vi "Dashboard Main20170221.vi"() -> ()   [LabVIEW 2016]
uses:
  <vilib>/Utility/miscctls.llb/LVRangeTypeDef.ctl
  <vilib>/Platform/TimedLoop/XDataNode/timing_clust.ctl
  <vilib>/Platform/TimedLoop/XDataNode/nitl_modes.ctl
  <vilib>/Platform/TimedLoop/XDataNode/wakeup.ctl
  <vilib>/Utility/miscctls.llb/LVRowAndColumnTypeDef.ctl
  <vilib>/event_ctls.llb/eventvkey.ctl
  <vilib>/Rock Robotics/WPI/Dashboard/WPI_DashboardLogging Global.vi
  <vilib>/Rock Robotics/Network Tables/NT Read Numeric Array.vi
  <vilib>/Rock Robotics/Network Tables/NT Write Boolean.vi
  <vilib>/platform/TimedLoop/XDataNode/XDataNode.xnode
  <vilib>/Platform/TimedLoop/XDataNode/XDNodeRunTimeDep.lvlib
panel:
  in  "Camera Tab":T1(tab)
  out "Image Message":string="Timeout in Camera Communications"
  in  "Camera Settings 1":T2={"Frame Rate"=30, "Compression"=30, "Size"=1, "DB Camera Config"=FALSE} {"Frame Rate" scale=1.0..30.0; "Compression" scale=100.0..-1.0; "Size" items=["640x480", "320x240", "160x120"]}
  out "Dashboard Image 1":T3(plugin-control)
  out "Camera Info 1":cluster{"Mbps LED":bool, "Mbps":dbl, "fps":dbl} {"fps" format="%#.1g"; "Mbps" format="%#.1g"}
  in  "Camera Name 1":string(combo)="No Camera Selection"
  out "Image Message 2":string="Timeout in Camera Communications"
  in  "Camera Settings 2":T2={"Frame Rate"=30, "Compression"=30, "Size"=1, "DB Camera Config"=FALSE} {"Frame Rate" scale=1.0..30.0; "Compression" scale=100.0..-1.0; "Size" items=["640x480", "320x240", "160x120"]}
  out "Dashboard Image 2":T3(plugin-control)
  out "Camera Info 2":cluster{"Mbps LED":bool, "Mbps":dbl, "fps":dbl} {"fps" format="%#.1g"; "Mbps" format="%#.1g"}
  in  "Camera Name 2":string(combo)="No Camera Selection"
  out "Image Message 3":string="Timeout in Camera Communications"
  in  "Camera Settings 3":T2={"Frame Rate"=30, "Compression"=30, "Size"=1, "DB Camera Config"=FALSE} {"Frame Rate" scale=1.0..30.0; "Compression" scale=100.0..-1.0; "Size" items=["640x480", "320x240", "160x120"]}
  out "Dashboard Image 3":T3(plugin-control)
  out "Camera Info 3":cluster{"Mbps LED":bool, "Mbps":dbl, "fps":dbl} {"fps" format="%#.1g"; "Mbps" format="%#.1g"}
  in  "Camera Name 3":string(combo)="No Camera Selection"
  out "Image 3":T3(plugin-control)
  out "Image 2":T3(plugin-control)
  out "Image":T3(plugin-control)
  in  "Graph Include Filter":string[](array[string])
  in  "Graph Exclude Filter":string[](array[string])
  in  "Combo Box 8":string(combo)
  in  "Combo Box 7":string(combo)
  in  "Combo Box 6":string(combo)
  in  "Combo Box 5":string(combo)
  in  "Combo Box 4":string(combo)
  in  "Combo Box 3":string(combo)
  in  "Combo Box 2":string(combo)
  in  "Combo Box":string(combo)
  out "Waveform Chart 2":dbl[][](graph)
  out "Waveform Chart":dbl[][](graph)
  in  "Pause":bool
  in  "# Samples":i32=20000
  in  "Reset":bool
  in  "TCP":refnum<k5>
  in  "Rec Mode":enum32{"Stop", "Record", "Playback"}(radio)
  out "Robot IP":string
  in  "Dashboard Tab":T4(tab)
  out "NT Connection":bool
  out "MotorChart R":cluster{"Numeric":dbl, "Numeric":dbl}(graph)
  out "MotorChart L":cluster{"Numeric":dbl, "Numeric":dbl}(graph)
  out "MotorSliders R":cluster{"MotorSlide1":dbl, "MotorSlide2":dbl} {"MotorSlide2" scale=-1.0..1.0 scale format="%#_2e"; "MotorSlide1" scale=-1.0..1.0 scale format="%#_2e"}
  out "MotorSliders L":cluster{"MotorSlide1":dbl, "MotorSlide2":dbl} {"MotorSlide2" scale=-1.0..1.0 scale format="%#_2e"; "MotorSlide1" scale=-1.0..1.0 scale format="%#_2e"}
  out "Gyro":dbl(knob) scale=0.0..360.0
  out "JS1 Z":dbl(slide) scale=-1.0..1.0 scale format="%#_2e"
  out "JS1 Graph":cluster{"X":dbl, "Y":dbl}[](graph)
  out "JS1 Buttons":T5
  out "JS2 Z":dbl(slide) scale=-1.0..1.0 scale format="%#_2e"
  out "JS2 Graph":cluster{"X":dbl, "Y":dbl}[](graph)
  out "JS2 Buttons":T5
  out "Mode":T6(ring)=enum."Auto Disabled"
  out "Background":bool
  in  "Get Data":bool
  in  "DB/String 9":string
  in  "DB/String 8":string
  in  "DB/String 7":string
  in  "DB/String 6":string
  in  "DB/String 5":string
  in  "DB/String 4":string
  in  "DB/String 3":string
  in  "DB/String 2":string
  in  "DB/String 1":string
  in  "DB/String 0":string
  in  "DB/Slider 0":dbl(slide) scale=0.0..5.0
  in  "DB/Slider 1":dbl(slide) scale=0.0..5.0
  in  "DB/Slider 2":dbl(slide) scale=0.0..5.0
  in  "DB/Slider 3":dbl(slide) scale=0.0..5.0
  out "DB/LED 3":bool
  out "DB/LED 2":bool
  out "DB/LED 1":bool
  out "DB/LED 0":bool
  in  "DB/Button 3":bool
  in  "DB/Button 2":bool
  in  "DB/Button 1":bool
  in  "DB/Button 0":bool caption="New Name"
  in  "Select Auto":string(combo)="Select Autonomous ..."
  in  "Select Test":string(combo)="Select Test ..."
  in  "Test Slider":dbl(slide) scale=0.0..100.0 scale format="%#_3g"
  in  "On/Off":bool caption="Solenoid"
  in  "Test Name":u16(ring) items=["Select the test to run..."]
  in  "Test Tree":string(tree)
  in  "Motor":cluster{"Value":dbl, "Enable":bool} {"Value" scale=-1.0..1.0 scale format="%#_3g"}
  out "Progress":T7 {"Test Progress" scale=0.0..100.0}
  in  "Rev/Fwd":cluster{"Forward":bool, "Reverse":bool}
  in  "Test Ring":u16(ring) items=["Monochrome", "Color"]
  out "Cmd Status":string
  in  "Execute Command":bool
  in  "Command Params":string[][](table)
  in  "Command Selection":i32(listbox)
  in  "CheckList":i32(listbox)
  out "Tree":string(tree)
  # "HW"
  # "HW"
  # "HW"
  # "Graph 1 Variable Selection"
  # "Graph 2 Variable Selection"
  # "Joysticks"
  # "Drive Motors"
  # "Front"
  # "Right"
  # "Left"
  # "Back"
  # "This tab is a great place for autonomous settings and robot-specific values.\nPlace controls and indicators inside this tab and match name to\nDashboard Variables on robot. You can also delete this comment."
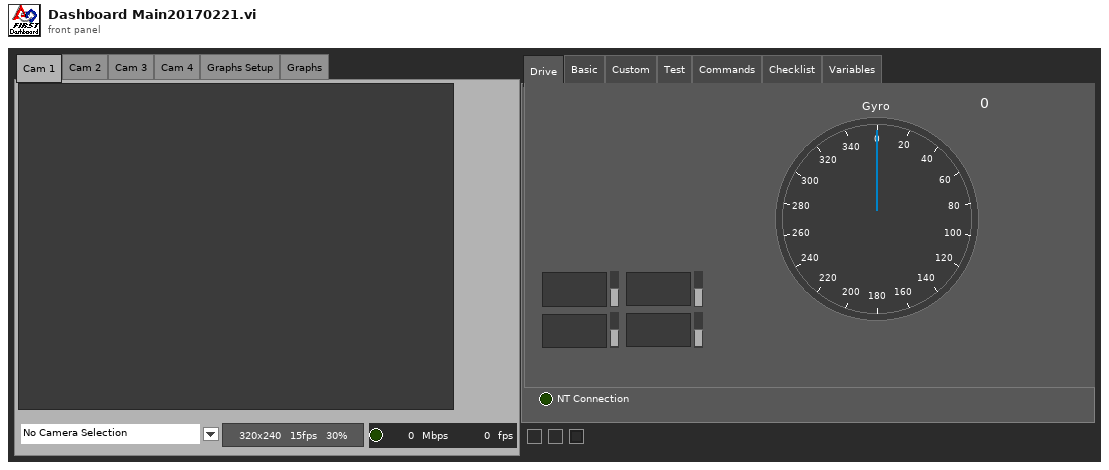
[diagram p1: front panel]
types:
  T1 = enum32{"Cam 1", "Cam 2", "Cam 3", "Cam 4", "Graphs Setup", "Graphs"}
  T2 = cluster{"Frame Rate":i32, "Compression":i32, "Size":u16, "DB Camera Config":bool}
  T3 = typedef "IMAQ Image.ctl" = refnum<image>
  T4 = enum32{"Drive", "Basic", "Custom", "Test", "Commands", "Checklist", "Variables"}
  T5 = cluster{bool, bool, bool, bool, bool, bool, bool, bool, bool, bool, bool, bool}
  T6 = enum8{"Tele-Op Disabled", "Tele-Op Enabled", "Auto Disabled", "Auto Enabled", "Test Disabled", "Test Enabled", "Disconnected", "No Code", "E-Stop"}
  T7 = cluster{"Test Progress":u8, "Test Progress Text":string}
  T8 = typedef "LVRangeTypeDef.ctl" = cluster{"Minimum":dbl, "Maximum":dbl, "Increment":dbl, "Minor Increment":dbl, "Start":dbl}
  T9 = cluster{"IDs":cluster{"RPC field ID":u16, "Unique ID":u16}, "String":string}
  T10 = enum32{"Drive", "Basic", "Custom", "Test", "Checklist", "Variables"}
  T11 = typedef "Image Type" = u32
  T12 = cluster{"Error Strings":string, "Disable Counts":cluster{u16, u16}, "Rail Faults":cluster{u16, u16, u16}, "Robot IP":string, "DB Mode":u8, "Event Info":cluster{"Name":string, "Type":u8, "Number":u16, "Replay":u8}}
  T13 = cluster{"Storage":cluster{"Disk Free":u64, "RAM Block":u32, "RAM free":u32}, "CPU Utilization":cluster{"CPU % ISR":sgl, "CPU % Time Crit":sgl, "CPU % Timed Str":sgl, "CPU % High":sgl, "CPU % Above":sgl, "CPU % Normal":sgl, "CPU % Low":sgl}, "CAN":cluster{"% Bus Utilization":sgl, "Bus Off Cnt":u32, "TX_FIFO Full Cnt":u32, "Receive Error Cnt":u8, "Transmit Error Cnt":u8}, "HID":cluster{"HID Outputs":u32, "Rumble Low":u16, "Rumble High":u16}[]}
  T14 = cluster{"Status bits":cluster{"Test Mode":bool, "Autonomous":bool, "Enabled":bool, "Code Start":bool, "Brownout":bool, "Reserved 2":bool, "Reserved 3":bool, "E-Stop":bool}, "Code Trace":cluster{"Disabled":bool, "TeleOp":bool, "Auto":bool, "Test":bool}, "Controller Type":enum16{"unknown", "cRIO", "roboRio"}, "Code?":enum16{"unknown", "noCode", "code"}, "Battery V":dbl}
  T15 = cluster{"Control Bits":cluster{"TestMode":bool, "Autonomous":bool, "Enabled":bool, "FMS Present":bool, bool, bool, bool, "E-Stop":bool}, "Team Station ":u8, "Countdown":sgl, "Joystick Values":cluster{"Axes":dbl[], "Buttons":bool[], "POVs":i16[]}[]}
  T16 = enum32{"Cam 1", "Cam 2", "Cam 3", "Cam 4", "Graphs Setup", "Graphs"}[]
  T17 = cluster{"Axes":dbl[], "Buttons":bool[], "POVs":i16[]}[]
  T18 = cluster{"Axes":dbl[], "Buttons":bool[], "POVs":i16[]}
  T19 = cluster{"Buttons[0]":bool, "Buttons[1]":bool, "Buttons[2]":bool, "Buttons[3]":bool, "Buttons[4]":bool, "Buttons[5]":bool, "Buttons[6]":bool, "Buttons[7]":bool, "Buttons[8]":bool, "Buttons[9]":bool, "Buttons[10]":bool, "Buttons[11]":bool}
  T20 = cluster{"Dashboard Image 1":refnum<vi>, "Dashboard Tab":refnum<vi>, "Background":refnum<vi>, "Rec Mode":refnum<vi>, "Test Slider":refnum<vi>, "On/Off ":refnum<vi>, "Test Ring":refnum<vi>, "Rev/Fwd":refnum<vi>, "Test Name":refnum<vi>, "Motor":refnum<vi>, "Progress":refnum<vi>, "CheckList":refnum<vi>, "Tree":refnum<vi>, "Test Tree":refnum<vi>, "Command Params":refnum<vi>, "Command Selection":refnum<vi>, "Execute Command":refnum<vi>, "Cmd Status":refnum<vi>, "Camera Settings 1":refnum<vi>, "Camera Name 1":refnum<vi>, "Camera Info 1":refnum<vi>, "Camera Settings 2":refnum<vi>, "Camera Name 2":refnum<vi>, "Dashboard Image 2":refnum<vi>, "Camera Tab":refnum<vi>, "Camera Info 2":refnum<vi>, "Dashboard Image 3":refnum<vi>, "Camera Settings 3":refnum<vi>, "Camera Name 3":refnum<vi>, "Camera Info 3":refnum<vi>, "Select Auto":refnum<vi>, "Select Test":refnum<vi>}
  T21 = cluster{"Operation":enum16{"Update", "Clear"}, "Color Box":u32}[]
  T22 = typedef "eventvkey.ctl" = enum16{"ASCII", "Enter", "Return", "Shift", "Ctrl", "Alt", "Cmd", "Opt", "Caps", "NumLock", "Clear", "Break", "Up", "Down", "Left", "Right", "Insert", "Delete", "Home", "End", "PageUp", "PageDown", "Escape", "Help", "Pause", "ScrollLock", "F1", "F2", "F3", "F4", "F5", "F6", "F7", "F8", "F9", "F10", "F11", "F12", "F13", "F14", "F15", "F16", "F17", "F18", "F19", "F20", "F21", "F22", "F23", "F24", "Play", "VolumeUp", "VolumeDown", "Mute", "Two Byte Char"}
  T23 = cluster{"Image Size":bool, "Image Type":bool, "Pixel Value":bool, "ROI Information":bool, "Zoom Factor":bool}
  T24 = cluster{"Operation":enum16{"Update", "Clear"}, "Color Box":u32}
  T25 = typedef "LVRowAndColumnTypeDef.ctl" = cluster{"Row":i32, "Column":i32}
  T26 = cluster{"Shift":bool, "Ctrl":bool, "Alt":bool, "Cmd":bool, "Opt":bool}
  T27 = typedef "XDNodeRunTimeDep.lvlib/timing_clust.ctl" = cluster{"Expected End [f-1]":u64, "Actual End [f-1]":u64, "Finished Late? [f-1]":bool, "Expected End [i-1]":u64, "Actual End [i-1]":u64, "Finished Late? [i-1]":bool, "Expected Start [i]":u64, "Actual Start [i]":u64, "Expected Start [f]":u64, "Actual Start [f]":u64, "Source Name":string, "Structure Name":string, "Period":i64, "Deadline":i64, "Offset":i64, "Start":i64, "Priority":i32, "Timeout":i32, "Mode":T28, "Wakeup Reason":T29, "Error":errorcluster, "Source Type":string, "Secondary Source Type":string, "Global End Time":u64, "Global Start Time":u64, "Frame Duration":u64, "Iteration Duration":u64, "Assigned CPU":i32, "I/O Scan Engine Mode":u32}
  T28 = typedef "XDNodeRunTimeDep.lvlib/nitl_modes.ctl" = enum32{"No Change", "Process missed periods, maintain original phase", "Discard missed periods, maintain original phase", "Process missed periods, ignore original phase", "Discard missed periods, ignore original phase"}
  T29 = typedef "XDNodeRunTimeDep.lvlib/wakeup.ctl" = enum32{"Normal", "Aborted", "Asynchronous wakeup", "Timing source error", "Timed loop error", "Timeout"}
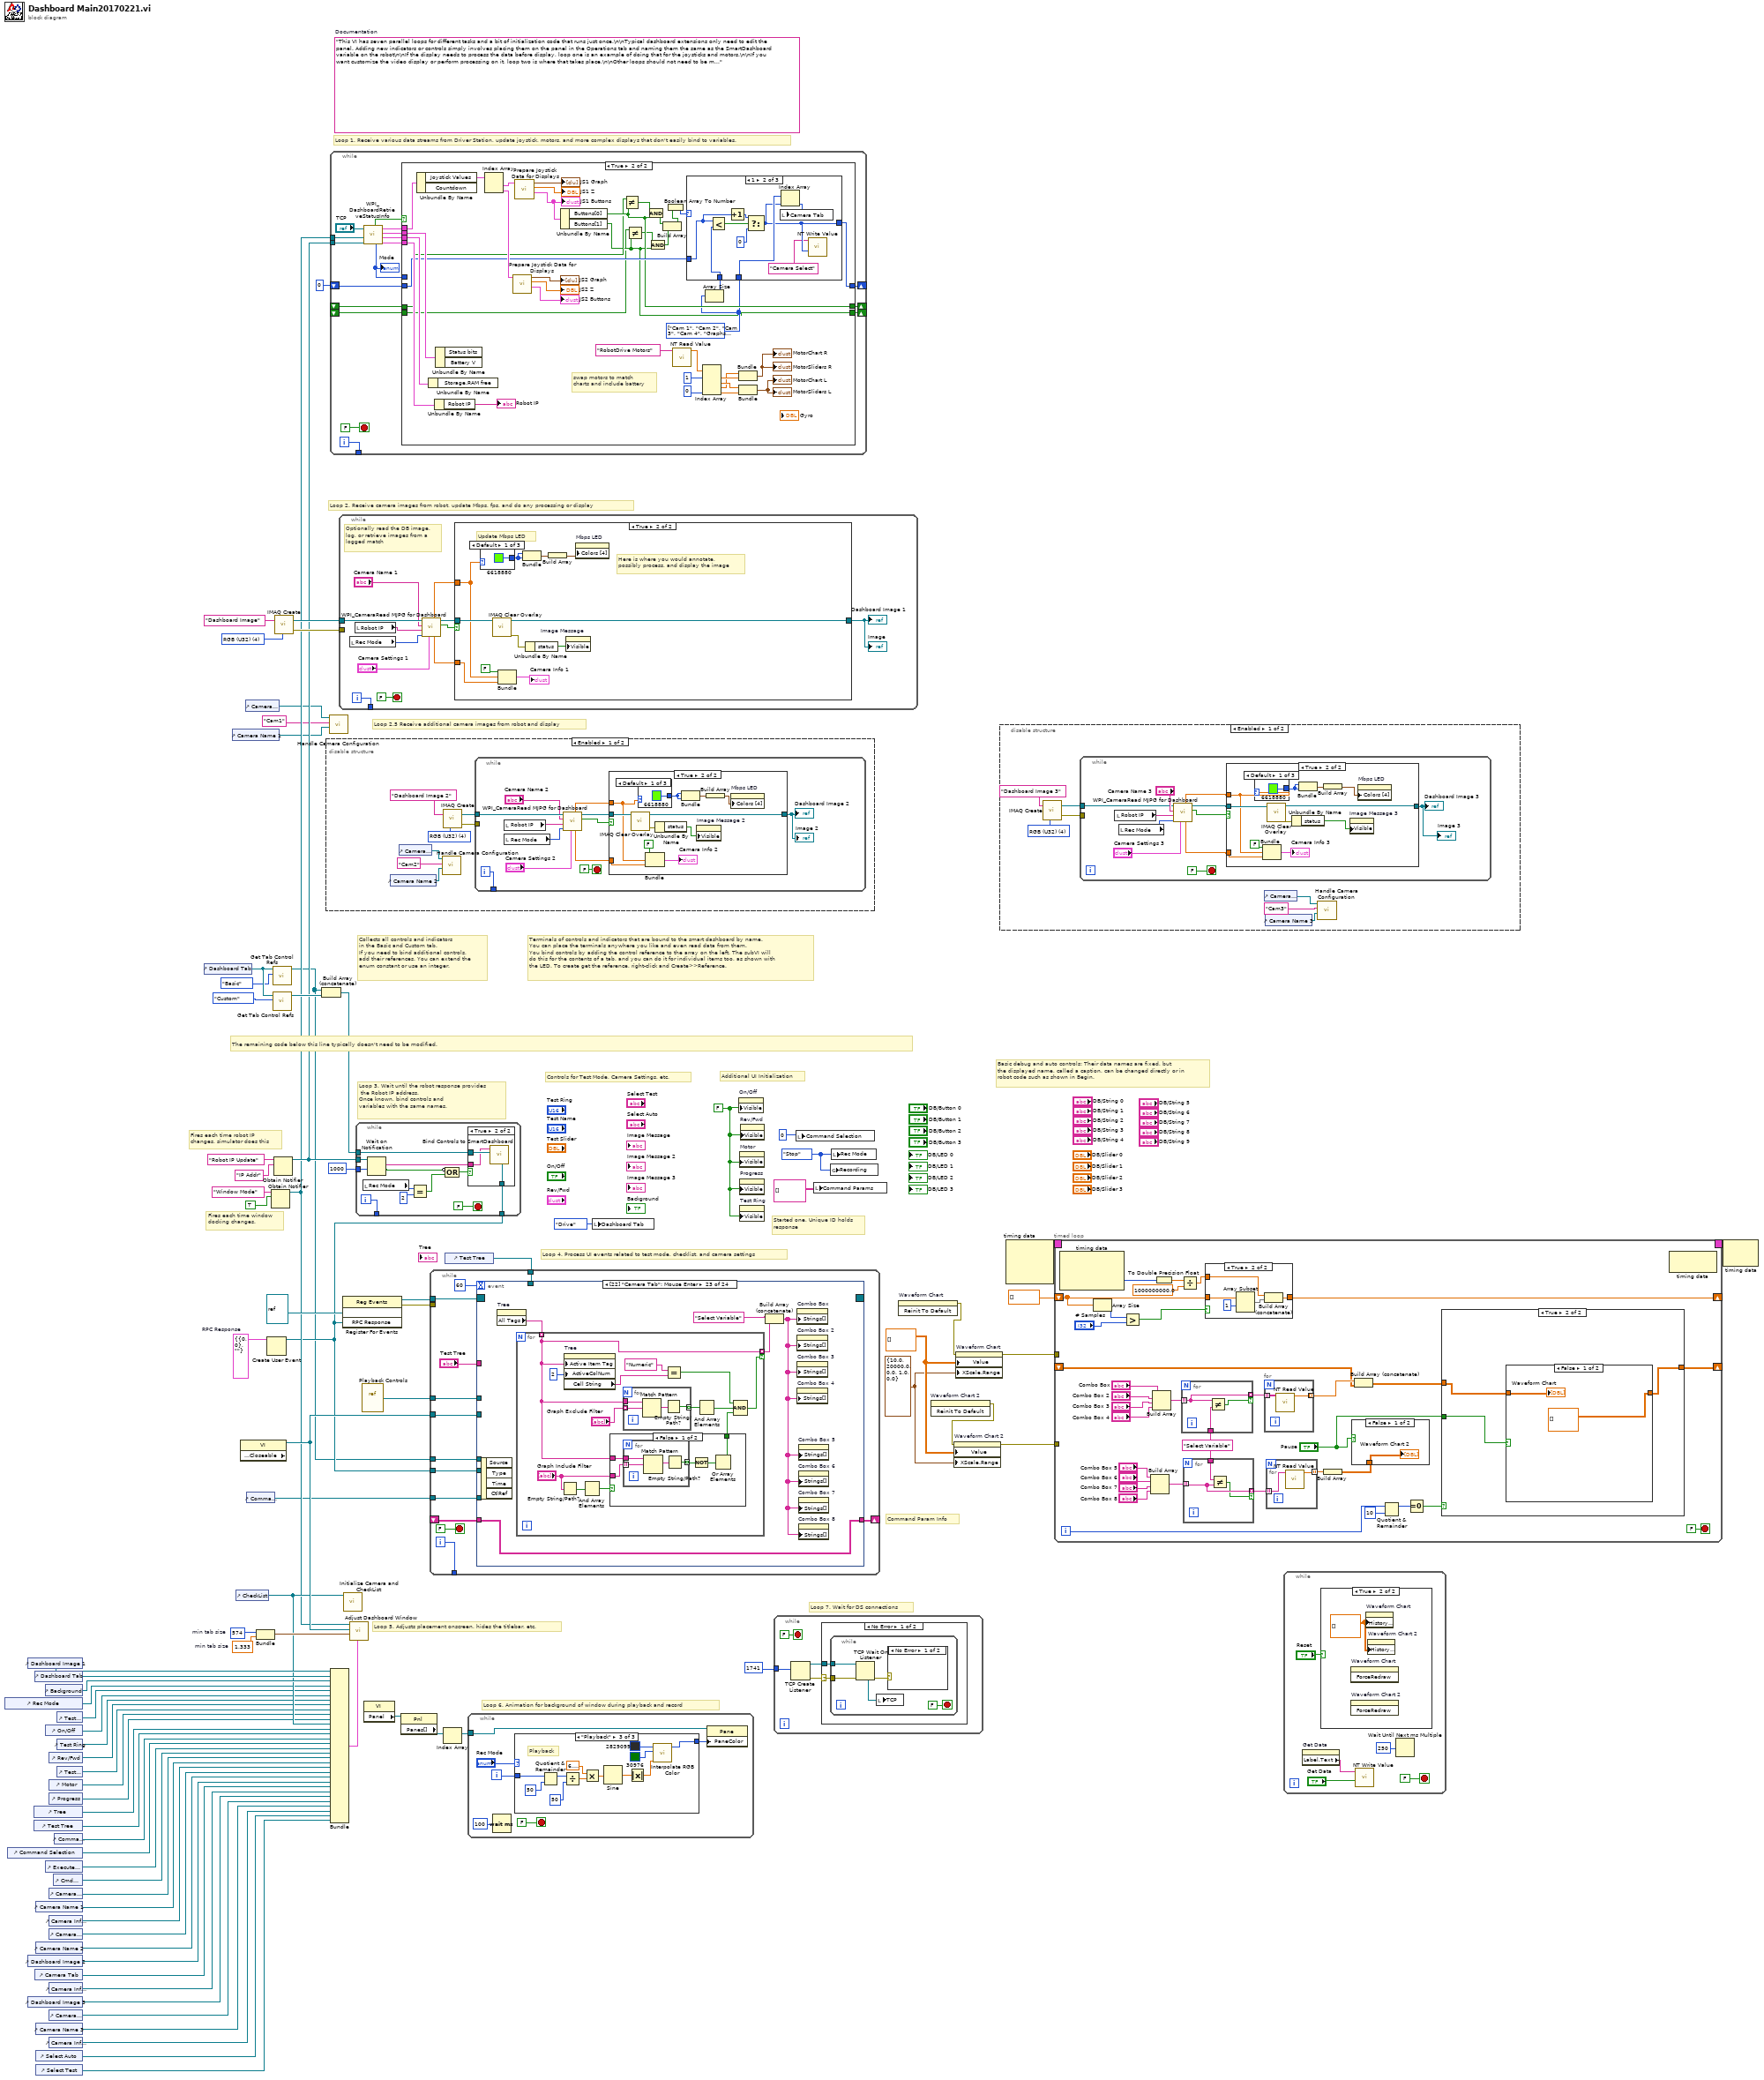
[diagram p0: block diagram]
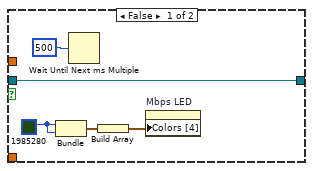
[diagram p3: hidden frame]
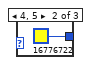
[diagram p4: hidden frame]
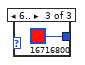
[diagram p5: hidden frame]
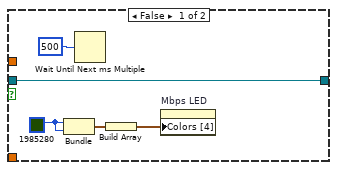
[diagram p7: hidden frame]
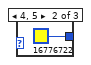
[diagram p8: hidden frame]
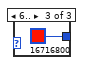
[diagram p9: hidden frame]
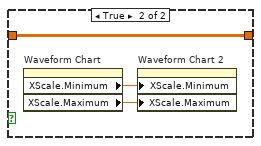
[diagram p13: hidden frame]
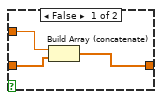
[diagram p14: hidden frame]
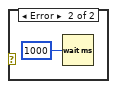
[diagram p15: hidden frame]
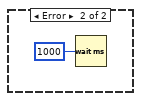
[diagram p16: hidden frame]
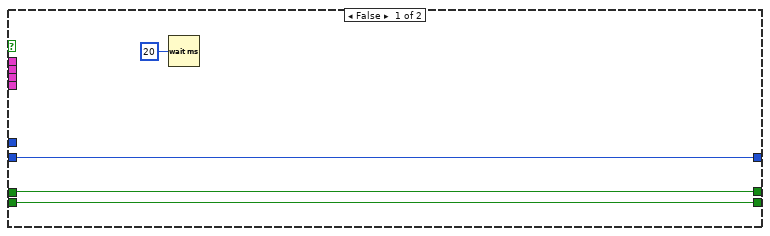
[diagram p17: hidden frame]
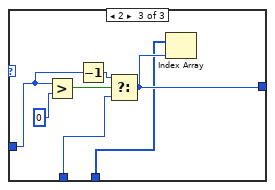
[diagram p19: hidden frame]
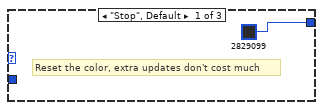
[diagram p20: hidden frame]
diagram:
  w3 = T8 {"Minimum"=10.0, "Maximum"=20000.0, "Increment"=0.0, "Minor Increment"=1.0, "Start"=0.0} ("X Scale.Range")
  w4 = dbl[][] [] ("Waveform Chart")
  w37 = T9 {"IDs"={"RPC field ID"=0, "Unique ID"=0}, "String"=""}  # RPC Response
  w60 = 574  # min tab size
  w59 = 1.333  # min tab size
  w67 = enum32{"Stop", "Record", "Playback"}."Stop" ("Rec Mode")
  w43 = FALSE ("Visible")
  (unwired) "This VI has seven parallel loops for different tasks and a bit of initialization code that runs just once.\n\nTypical dashboard extensions only need to edit the panel. Adding new indicators or controls simply involves placing them on the panel in the Operations tab and naming them the same as the SmartDashboard variable on the robot\n\nIf the display needs to process the data before display, loop one is an example of doing that for the joysticks and motors.\n\nIf you want customize the video display or perform processing on it, loop two is where that takes place.\n\nOther loops should not need to be modified. They are pretty standard, and document the task they perform."  # Documentation
  w84 = T11 4 items=["Grayscale (U8)", "Grayscale (I16)", "Grayscale (SGL)", "Complex (CSG)", "RGB (U32)", "HSL (U32)", "RGB (U64)"] ("Image Type")
  # "Loop 2.5 Receive additional camera images from robot and display"
  # "Command Param Info"
  # "Started one, Unique ID holds\nresponse"
  # "Loop 7. Wait for DS connections"
  # "Basic debug and auto controls: Their data names are fixed, but\nthe displayed name, called a caption, can be changed directly or in\nrobot code such as shown in Begin."
  # "Controls for Test Mode, Camera Settings, etc."
  # "Additional UI Initialization"
  # "Loop 6. Animation for background of window during playback and record"
  # "Fires each time robot IP\nchanges, simulator does this"
  # "Fires each time window\ndocking changes."
  # "Collects all controls and indicators\nin the Basic and Custom tab.\nIf you need to bind additional controls,\nadd their references. You can extend the\nenum constant or use an integer."
  # "The remaining code below this line typically doesn't need to be modified."
  # "Loop 4. Process UI events related to test mode, checklist, and camera settings"
  # "Terminals of controls and indicators that are bound to the smart dashboard by name.\nYou can place the terminals anywhere you like and even read data from them.\nYou bind controls by adding the control reference to the array on the left. The subVI will\ndo this for the contents of a tab, and you can do it for individual items too, as shown with\nthe LED. To create get the reference, right-click and Create>>Reference."
  # "Loop 3. Wait until the robot response provides\n the Robot IP address.\nOnce known, bind controls and\nvariables with the same names."
  # "Loop 5. Adjusts placement onscreen, hides the titlebar, etc."
  # "Loop 1. Receive various data streams from Driver Station, update joystick, motors, and more complex displays that don't easily bind to variables."
  # "Loop 2. Receive camera images from robot, update Mbps, fps, and do any processing or display"
  n1 = control-ref of="Rec Mode"() -> (w49:refnum<vi>)
  n2 = control-ref of="Command Selection"() -> (w36:refnum<vi>)
  n3 = control-ref of="Dashboard Image 1"() -> (w62:refnum<vi>)
  n4 = control-ref of="Dashboard Image 2"() -> (w23:refnum<vi>)
  n5 = control-ref of="Dashboard Image 3"() -> (w13:refnum<vi>)
  n6 = control-ref of="Tree"() -> (w53:refnum<vi>)
  n7 = control-ref of="Test Tree"() -> (w52:refnum<vi>)
  n8 = control-ref of="Dashboard Tab"() -> (w61:refnum<vi>)
  n9 = control-ref of="Camera Tab"() -> (w21:refnum<vi>)
  n10 = control-ref of="Camera Name 1"() -> (w17:refnum<vi>)
  n11 = control-ref of="Camera Name 2"() -> (w16:refnum<vi>)
  n12 = control-ref of="Camera Name 3"() -> (w11:refnum<vi>)
  n13 = control-ref of="Select Auto"() -> (w9:refnum<vi>)
  n14 = control-ref of="Select Test"() -> (w8:refnum<vi>)
  n15 = control-ref of="Background"() -> (w57:refnum<vi>)
  n16 = control-ref of="On/Off"() -> (w47:refnum<vi>)
  n17 = control-ref of="Execute Command"() -> (w38:refnum<vi>)
  n18 = control-ref of="Rev/Fwd"() -> (w45:refnum<vi>)
  n19 = control-ref of="Motor"() -> (w50:refnum<vi>)
  n20 = control-ref of="Progress"() -> (w44:refnum<vi>)
  n21 = control-ref of="Camera Settings 1"() -> (w28:refnum<vi>)
  n22 = control-ref of="Camera Info 1"() -> (w27:refnum<vi>)
  n23 = control-ref of="Camera Settings 2"() -> (w24:refnum<vi>)
  n24 = control-ref of="Camera Info 2"() -> (w19:refnum<vi>)
  n25 = control-ref of="Camera Settings 3"() -> (w12:refnum<vi>)
  n26 = control-ref of="Camera Info 3"() -> (w10:refnum<vi>)
  n27 = control-ref of="Cmd Status"() -> (w32:refnum<vi>)
  n28 = control-ref of="Command Params"() -> (w39:refnum<vi>)
  n29 = control-ref of="Test Slider"() -> (w48:refnum<vi>)
  n30 = control-ref of="Test Ring"() -> (w46:refnum<vi>)
  n31 = control-ref of="Test Name"() -> (w51:refnum<vi>)
  n32 = control-ref of="Dashboard Tab"() -> (w65:refnum<vi>)
  n33 = control-ref of="Camera Name 1"() -> (w29:refnum<vi>)
  n34 = control-ref of="CheckList"() -> (w54:refnum<vi>)
  n35 = property class="VI" props=["Front Panel.Closeable"]() -> (reference out=w66:refnum<vi>)  [unwired: 2 in, 2 out]
  n36 = control-ref of="Camera Settings 1"() -> (w30:refnum<vi>)
  n37 = control-ref of="Command Params"() -> (w31:refnum<vi>)
  n38 = Bundle("min tab size"=w60, "min tab size"=w59) -> (w58:cluster{"min tab size":i32, "min tab size":dbl})  [unwired: 1 in]
  n39 = Create User Event(user event datatype=w37) -> (user event=w33:refnum<user-event>)  [unwired: 1 in, 1 out]
  n40 = Obtain Notifier(name (unnamed)="Window Mode", notification data type=TRUE) -> (notifier out=w41:refnum<notifier>)  [unwired: 2 in, 2 out]
  n41 = call <vilib>:"Get Tab Control Refs.vi"("Page Index"=T10."Basic" ("Dashboard Tab"), "TabControl in"=w65) -> ("ControlsOnPage"=w26:refnum<vi>[])  [unwired: 9 in]
  n42 = call <vilib>:"Get Tab Control Refs.vi"("Page Index"=T10."Custom" ("Dashboard Tab"), "TabControl in"=w65) -> ("ControlsOnPage"=w64:refnum<vi>[])  [unwired: 9 in]
  n43 = Obtain Notifier(name (unnamed)="Robot IP Update", notification data type="IP Addr" ("name (unnamed)")) -> (notifier out=w42:refnum<notifier>)  [unwired: 2 in, 2 out]
  n44 = call "IMAQ Create"("Image Name"="Dashboard Image", "Image Type"=w84) -> ("New Image"=w82:T3, "error out"=w81:errorcluster)  [unwired: 2 in, 1 out]
  n45 = Build Array (concatenate)(w26, w64) -> (w63:refnum<vi>[])
  n46 = disable-structure shown="Enabled" {
    frame Enabled {
      w86 = T11 4 items=["Grayscale (U8)", "Grayscale (I16)", "Grayscale (SGL)", "Complex (CSG)", "RGB (U32)", "HSL (U32)", "RGB (U64)", "Grayscale (U16)"] ("Image Type")
      n47 = control-ref of="Camera Name 2"() -> (w88:refnum<vi>)
      n48 = control-ref of="Camera Settings 2"() -> (w89:refnum<vi>)
      n49 = call "Handle Camera Configuration.vi"("CameraNameRef"=w88, "Camera File Name"="Cam2", "ClusterRef"=w89) -> ()  [unwired: 9 in]
      n50 = call "IMAQ Create"("Image Name"="Dashboard Image 2", "Image Type"=w86) -> ("New Image"=w85:T3, "error out"=w90:errorcluster)  [unwired: 2 in, 1 out]
      n51 = while {
        tunnel: w85 -> [w97]
        tunnel: w90 -> [_]
        tunnel: [w101] -> _
        i -> [w101]
        stop <- FALSE stop-if-true
        n52 = local read "Robot IP"() -> (w95:string)
        n53 = local read "Rec Mode"() -> (w94:enum32{"Stop", "Record", "Playback"})
        n54 = call <vilib>:"WPI_CameraRead MJPG for Dashboard.vi"("Camera Settings"="Camera Settings 2", "Rec Mode"=w94, "Robot IP"=w95, "Camera Name"="Camera Name 2", "Refnum in"=w97) -> ("Active"=w100:bool, "Refnum out"=w103:T3, "FPS"=w98:dbl, "Bandwidth (Mbps)"=w99:dbl)  [unwired: 3 in]
        n55 = case shown="True" w100 {
          tunnel: w103 -> [w107 w117]
          tunnel: w99 -> [_ w113]
          tunnel: w98 -> [_ w118]
          tunnel: [w107 w116] -> w92
          frame False {
            w105 = u32 1985280 ("Color Box")
            n56 = Bundle("Color Box"=w105, "Color Box"=w105) -> (w104:cluster{"Color Box":u32, "Color Box":u32})  [unwired: 1 out]
            n57 = Wait Until Next ms Multiple(millisecond multiple=u32 500) -> ()  [unwired: 1 out]
            n58 = Build Array(w104) -> (w106:cluster{"Color Box":u32, "Color Box":u32}[])
            n59 = property on="Mbps LED" class="Bool (strict)"("Colors [4]"=w106) -> ()  [unwired: 2 in, 2 out]
          }
          frame True {
            n60 = call "IMAQ Clear Overlay"("Image"=w117) -> ("error out"=w115:errorcluster, "Image Out"=w116:T3)  [unwired: 2 in, 7 out]
            n61 = case shown="Default" w113 {
              tunnel: [u32 6618880 ("Color Box") u32 16776722 ("Color Box") u32 16716800 ("Color Box")] -> w111
              frame Default {
              }
              frame 4, 5 {
              }
              frame 6.. {
              }
            }
            n62 = Bundle(FALSE, "Bandwidth (Mbps)"=w113, "FPS"=w118) -> (→"Camera Info 2":cluster{bool, "Bandwidth (Mbps)":dbl, "FPS":dbl})  [unwired: 1 in]
            n63 = Unbundle By Name(w115) -> ("status"=w114:bool)
            n64 = Bundle("Color Box"=w111, "Color Box"=w111) -> (w112:cluster{"Color Box":u32, "Color Box":u32})  [unwired: 1 out]
            n65 = property on="Image Message 2" class="Str"("Visible"=w114) -> ()  [unwired: 2 in, 2 out]
            n66 = Build Array(w112) -> (w110:cluster{"Color Box":u32, "Color Box":u32}[])
            n67 = property on="Mbps LED" class="Bool (strict)"("Colors [4]"=w110) -> ()  [unwired: 2 in, 2 out]
          }
        }
        "Dashboard Image 2" <- w92
        "Image 2" <- w92
      }
    }
    frame Disabled {
    }
  }
  n68 = call "Handle Camera Configuration.vi"("CameraNameRef"=w29, "Camera File Name"="Cam1", "ClusterRef"=w30) -> ()  [unwired: 9 in]
  n69 = while {
    tunnel: [w138] -> _
    tunnel: w42 -> [w132]
    tunnel: w41 -> [w129]
    shift-right: [w127] -> _
    shift-left: 0 ("index") -> [w128]
    shift-right: [w126] -> _
    shift-left: _ -> [w125]
    shift-right: [w124] -> _
    shift-left: _ -> [w123]
    i -> [w138]
    stop <- FALSE stop-if-true
    n70 = call <vilib>:"WPI_DashboardRetrieveStatusInfo.vi"("Binding Refnum"=w132, "Window Mode Notifier"=w129, "TCP Cnx"="TCP") -> ("Power and Errors"=w133:T12, "Robot Metrics"=w136:T13, "Status Info"=w137:T14, "Control Info"=w134:T15, "Robot Mode"=w131:T6, "Process?"=w135:bool)  [unwired: 3 in]
    "Mode" <- w131
    n71 = case shown="True" w135 {
      tunnel: w137 -> [_ w181]
      tunnel: w136 -> [_ w180]
      tunnel: w134 -> [_ w179]
      tunnel: w133 -> [_ w178]
      tunnel: w131 -> [_ _]
      tunnel: w128 -> [w142 w157]
      tunnel: [w142 w156] -> w127
      tunnel: [w141 w154] -> w126
      tunnel: w125 -> [w141 w153]
      tunnel: [w140 w149] -> w124
      tunnel: w123 -> [w140 w148]
      frame False {
        n72 = Wait (ms)(milliseconds to wait=u32 20) -> ()  [unwired: 1 out]
      }
      frame True {
        w152 = T16 [enum."Cam 1", enum."Cam 2", enum."Cam 3", enum."Cam 4", enum."Graphs Setup", enum."Graphs"] items=["Cam 1", "Cam 2", "Cam 3", "Cam 4", "Graphs Setup", "Graphs"]
        # "swap motors to match\ncharts and include battery"
        n73 = Unbundle By Name(w179) -> ("Joystick Values"=w169:T17)  [unwired: 1 out]
        n74 = Unbundle By Name(w180) -> ()  [unwired: 1 out]
        n75 = Unbundle By Name(w178) -> ("Robot IP"=→"Robot IP":string)
        n76 = Unbundle By Name(w181) -> ()  [unwired: 2 out]
        n77 = Index Array(array=w169) -> (element #1=w168:T18, element #2=w165:T18)  [unwired: 2 in]
        n78 = call "Prepare Joystick Data for Displays.vi"("Joystick Values"=w165) -> ("Buttons"=→"JS2 Buttons":T19, "Z Axis"=→"JS2 Z":dbl, "Cartesian Data"=→"JS2 Graph":cluster{"X axis":dbl, "X axis":dbl}[])  [unwired: 8 in]
        n79 = call "Prepare Joystick Data for Displays.vi"("Joystick Values"=w168) -> ("Buttons"=w158:T19, "Z Axis"=→"JS1 Z":dbl, "Cartesian Data"=→"JS1 Graph":cluster{"X axis":dbl, "X axis":dbl}[])  [unwired: 8 in]
        "JS1 Buttons" <- w158
        n80 = Unbundle By Name(w158) -> ("Buttons[0]"=w154:bool, "Buttons[1]"=w149:bool)
        n81 = Not Equal?(x=w153, y=w154) -> (x != y?=w155:bool)
        n82 = Not Equal?(x=w148, y=w149) -> (x != y?=w150:bool)
        n83 = And(x=w155, y=w154) -> (x .and. y?=w147:bool)
        n84 = And(x=w150, y=w149) -> (x .and. y?=w146:bool)
        n85 = Build Array(w147, w146) -> (w145:bool[])
        n86 = Boolean Array To Number(Boolean array=w145) -> (number=w144:u32)
        n87 = call-poly <vilib>:"NT Read Value.vi"("Name"="RobotDrive Motors") -> ("Numeric Array"=w160:dbl[])  [unwired: 9 in, 1 out]
        n88 = Index Array(array=w160, index #1=1, index #4=0) -> (element #1=w173:dbl, element #2=w174:dbl, element #3=w172:dbl, element #4=w177:dbl)  [unwired: 2 in]
        n89 = Array Size(array=w152) -> (size(s)=w151:i32)
        n90 = case shown="1" w144 {
          tunnel: w152 -> [_ w187 w195]
          tunnel: w157 -> [w182 w186 w194]
          tunnel: [w182 w184 w196] -> w156
          tunnel: w151 -> [_ w185 w193]
          frame 0, Default {
          }
          frame 1 {
            n91 = Less?(x=w186, y=w185) -> (x < y?=w191:bool)
            n92 = Increment(x=w186) -> (x+1=w190:i32)
            n93 = Select(t=w190, s=w191, f=0) -> (s? t:f=w184:i32)
            n94 = Index Array(array=w187, index=w184) -> (element=w188:T1)
            n95 = local write "Camera Tab"(w188) -> ()
            n96 = call-poly <vilib>:"NT Write Value.vi"("Numeric"=w184, "Name"="Camera Select") -> ()  [unwired: 9 in, 1 out]
          }
          frame 2 {
            n97 = Greater?(x=w194, y=0) -> (0:w198:bool)
            n98 = Decrement(x=w194) -> (x-1=w197:i32)
            n99 = Select(t=w197, s=w198, f=w193) -> (s? t:f=w196:i32)
            n100 = Index Array(array=w195, index=w196) -> ()  [unwired: 1 out]
          }
        }
        n101 = Bundle("Numeric"=w172, "Numeric"=w173) -> (→"MotorChart R" →"MotorSliders R":cluster{"Numeric":dbl, "Numeric":dbl})  [unwired: 1 in]
        n102 = Bundle("Numeric"=w174, "Numeric"=w177) -> (→"MotorChart L" →"MotorSliders L":cluster{"Numeric":dbl, "Numeric":dbl})  [unwired: 1 in]
      }
    }
  }
  n103 = Bundle("Dashboard Image 1"=w62, "Dashboard Tab"=w61, "Background"=w57, "Rec Mode"=w49, "Test Slider"=w48, "On/Off"=w47, "Test Ring"=w46, "Rev/Fwd"=w45, "Test Name"=w51, "Motor"=w50, "Progress"=w44, "CheckList"=w54, "Tree"=w53, "Test Tree"=w52, "Command Params"=w39, "Command Selection"=w36, "Execute Command"=w38, "Cmd Status"=w32, "Camera Settings 1"=w28, "Camera Name 1"=w17, "Camera Info 1"=w27, "Camera Settings 2"=w24, "Camera Name 2"=w16, "Dashboard Image 2"=w23, "Camera Tab"=w21, "Camera Info 2"=w19, "Dashboard Image 3"=w13, "Camera Settings 3"=w12, "Camera Name 3"=w11, "Camera Info 3"=w10, "Select Auto"=w9, "Select Test"=w8) -> (w20:T20)  [unwired: 1 in]
  n104 = while {
    tunnel: w82 -> [w208]
    tunnel: w81 -> [_]
    tunnel: [w209] -> _
    i -> [w209]
    stop <- FALSE stop-if-true
    # "Optionally read the DB image,\nlog, or retrieve images from a\nlogged match"
    n105 = local read "Rec Mode"() -> (w204:enum32{"Stop", "Record", "Playback"})
    n106 = local read "Robot IP"() -> (w203:string)
    n107 = call <vilib>:"WPI_CameraRead MJPG for Dashboard.vi"("Camera Settings"="Camera Settings 1", "Rec Mode"=w204, "Robot IP"=w203, "Camera Name"="Camera Name 1", "Refnum in"=w208) -> ("Active"=w206:bool, "Refnum out"=w207:T3, "FPS"=w205:dbl, "Bandwidth (Mbps)"=w202:dbl)  [unwired: 3 in]
    n108 = case shown="True" w206 {
      tunnel: w207 -> [w211 w222]
      tunnel: w202 -> [_ w219]
      tunnel: w205 -> [_ w220]
      tunnel: [w211 w216] -> w199
      frame False {
        w213 = u32 1985280 ("Color Box")
        # "Sleep for 500ms"
        n109 = Bundle("Color Box"=w213, "Color Box"=w213) -> (w214:cluster{"Color Box":u32, "Color Box":u32})  [unwired: 1 out]
        n110 = Build Array(w214) -> (w212:cluster{"Color Box":u32, "Color Box":u32}[])
        n111 = property on="Mbps LED" class="Bool (strict)"("Colors [4]"=w212) -> ()  [unwired: 2 in, 2 out]
        n112 = Wait Until Next ms Multiple(millisecond multiple=u32 500) -> ()  [unwired: 1 out]
      }
      frame True {
        # "Here is where you would annotate,\npossibly process, and display the image"
        # "Update Mbps LED"
        n113 = case shown="Default" w219 {
          tunnel: [u32 6618880 ("Color Box") u32 16776722 ("Color Box") u32 16716800 ("Color Box")] -> w223
          frame Default {
          }
          frame 4, 5 {
          }
          frame 6.. {
          }
        }
        n114 = call "IMAQ Clear Overlay"("Image"=w222) -> ("error out"=w225:errorcluster, "Image Out"=w216:T3)  [unwired: 2 in, 7 out]
        n115 = Bundle(FALSE, "Bandwidth (Mbps)"=w219, "FPS"=w220) -> (→"Camera Info 1":cluster{bool, "Bandwidth (Mbps)":dbl, "FPS":dbl})  [unwired: 1 in]
        n116 = Bundle("Color Box"=w223, "Color Box"=w223) -> (w224:cluster{"Color Box":u32, "Color Box":u32})  [unwired: 1 out]
        n117 = Unbundle By Name(w225) -> ("status"=w226:bool)
        n118 = Build Array(w224) -> (w221:cluster{"Color Box":u32, "Color Box":u32}[])
        n119 = property on="Image Message" class="Str"("Visible"=w226) -> ()  [unwired: 2 in, 2 out]
        n120 = property on="Mbps LED" class="Bool (strict)"("Colors [4]"=w221) -> ()  [unwired: 2 in, 2 out]
      }
    }
    "Dashboard Image 1" <- w199
    "Image" <- w199
  }
  n121 = register-events(refnum<vi> refnum, w33) -> (reference out=w71:refnum<event-registration>, error out=w70:errorcluster)  [unwired: 2 in]
  n122 = call "Initialize Camera and CheckList.vi"("ListBox in"=w54) -> ()  [unwired: 11 in]
  n123 = call "Adjust Dashboard Window.vi"("Sizing Refnums"=w20, "Size Constraints"=w58, "VI"=w66, "WIn Mode"=w41) -> ()  [unwired: 8 in]
  n124 = while {
    tunnel: w63 -> [w241]
    tunnel: w42 -> [w239]
    tunnel: [w237] -> _
    tunnel: u32 1000 ("milliseconds to wait") -> [w236]
    tunnel: w33 -> [w230]
    i -> [w237]
    stop <- FALSE stop-if-true
    n125 = local read "Rec Mode"() -> (w232:enum32{"Stop", "Record", "Playback"})
    n126 = Wait on Notification(notifier=w239, timeout in ms (-1)=w236) -> (notification=w238:string, timed out?=w234:bool)  [unwired: 2 in, 2 out]
    n127 = Equal?(x=w232, y=u16 2 ("Rec Mode")) -> (x = y?=w233:bool)
    n128 = Compound Arithmetic op=OR(invert w234, w233) -> (w235:bool)
    n129 = case shown="True" w235 {
      tunnel: w241 -> [_ w244]
      tunnel: w238 -> [_ w243]
      tunnel: w230 -> [_ w242]
      frame False {
      }
      frame True {
        n130 = call <vilib>:"Bind Controls to SmartDashboard.vi"("RPC ref"=w242, "Bound Control Refs"=w244, "Server IP Address"=w243) -> ()  [unwired: 9 in]
      }
    }
  }
  n131 = vi-ref "Playback Controls.vi"() -> (w72:refnum<vi>)
  n132 = property class="VI"() -> ("Panel"=w74:refnum<vi>)  [unwired: 2 in, 2 out]
  n133 = property class="Pnl"(reference=w74) -> ("Panes[]"=w75:refnum<vi>[])  [unwired: 1 in, 2 out]
  n134 = Index Array(array=w75) -> (element=w73:refnum<vi>)  [unwired: 1 in]
  n135 = control-ref of="Test Tree"() -> (w76:refnum<vi>)
  n136 = while {
    tunnel: [w254] -> _
    tunnel: w76 -> [w253]
    tunnel: w72 -> [w252]
    tunnel: w71 -> [w251]
    tunnel: w70 -> [_]
    tunnel: w66 -> [w250]
    tunnel: w33 -> [w249]
    tunnel: w31 -> [w248]
    shift-right: [w247] -> _
    shift-left: _ -> [w246]
    tunnel: w26 -> [w245]
    i -> [w254]
    stop <- FALSE stop-if-true
    n137 = event shown="[22] \"Camera Tab\": Mouse Enter" {
      selector: w251 -> [_ _ _ _ _ _ _ _ _ _ _ _ _ _ _ _ _ _ _ _ _ _ _ _]
      dyn-events: [_ _ _ _ _ _ _ _ _ _ _ _ _ _ _ _ _ _ w518 _ _ _ _ _] -> _
      timeout: u32 60 ("milliseconds to wait") -> [_ _ _ _ _ _ _ _ _ _ _ _ _ _ _ _ _ _ _ _ _ _ _ _]
      tunnel: w253 -> [w267 _ _ _ _ _ _ _ _ _ _ _ _ _ _ _ _ _ _ _ _ _ _ _]
      tunnel: "Test Tree" -> [_ _ _ _ _ _ _ _ _ _ _ _ _ w485 w493 w495 w499 w507 _ _ _ _ _ _]
      tunnel: w252 -> [_ _ _ _ _ _ _ _ _ _ _ _ _ _ _ _ _ _ w520 _ w538 _ _ _]
      tunnel: w250 -> [_ _ _ _ _ _ _ _ _ _ _ _ _ _ _ _ _ _ w516 _ _ _ _ _]
      tunnel: w249 -> [_ _ _ _ _ _ _ _ _ _ _ _ _ _ _ _ _ _ w512 _ _ _ _ _]
      tunnel: w248 -> [w262 _ _ _ _ _ _ _ w436 _ _ _ _ _ _ _ _ _ _ _ _ _ _ _]
      tunnel: [w261 w307 w409 w414 w423 w427 w430 w433 w434 w443 w453 w460 w472 w484 w491 w494 w498 w506 w511 w533 w535 w539 w548 w582] -> w247
      tunnel: w246 -> [w261 w307 w409 w414 w423 w427 w430 w433 w434 _ _ w460 w472 w484 w491 w494 w498 w506 w511 w533 w535 w539 w548 w582]
      tunnel: w245 -> [w259 _ _ _ _ _ _ _ _ _ _ _ _ _ _ _ _ _ _ _ _ _ _ _]
      event Timeout {
        n138 = event-data() -> ()  [unwired: 1 in, 1 out]
        n139 = call <vilib>:"Connextion Info.vi"() -> ("Connected"=→"NT Connection":bool)  [unwired: 10 in, 1 out]
        n140 = local read "Mode"() -> (w264:T6)
        n141 = case shown="\"Test\"" "Dashboard Tab" {
          tunnel: w267 -> [_ _ w283 _ _]
          tunnel: "/TestMode/Automatic/" ("Name Pattern") -> [_ _ w282 _ _]
          tunnel: T21 [{"Operation"=enum."Clear", "Color Box"=14013909}, {"Operation"=enum."Clear", "Color Box"=14013909}, {"Operation"=enum."Clear", "Color Box"=14013909}, {"Operation"=enum."Clear", "Color Box"=14013909}, {"Operation"=enum."Update", "Color Box"=14013909}, {"Operation"=enum."Update", "Color Box"=16777215}, {"Operation"=enum."Clear", "Color Box"=14013909}, {"Operation"=enum."Clear", "Color Box"=14013909}, {"Operation"=enum."Clear", "Color Box"=14013909}] -> [_ _ w275 _ w300]
          tunnel: w264 -> [_ _ w274 _ w299]
          tunnel: u32[] [15790320, 15790320, 15790320, 15790320, 16777215, 16777215, 15790320, 15790320, 15790320] -> [_ _ _ _ w305]
          tunnel: w262 -> [_ _ _ _ w293]
          tunnel: w259 -> [_ w269 _ _ _]
          frame "Custom", Default {
          }
          frame "Basic" {
            n142 = call <vilib>:"WPI_DashboardUpdateNames.vi"("Controls on Tab"=w269) -> ()  [unwired: 11 in]
          }
          frame "Test" {
            w281 = -2 ("Active Item:Row Number")
            n143 = Index Array(array=w275, index=w274) -> (element=w276:T24)
            n144 = Unbundle(w276) -> ("Operation"=w277:enum16{"Update", "Clear"}, "Color Box"=w278:u32)
            n145 = call <vilib>:"NT Read String.vi"("Name"="/TestMode/TestName") -> ("String"=w272:string)  [unwired: 9 in, 1 out]
            n146 = call <vilib>:"NT Read and Format Entries as Tree.vi"("Operation"=w277, "Name Pattern"=w282, "Tree Refnum"=w283) -> ()  [unwired: 7 in, 2 out]
            n147 = case shown="Default" w272 {
              tunnel: "/TestMode/TestProgress" ("Name") -> [w285 _]
              tunnel: "/TestMode/TestProgressText" ("Name") -> [w284 _]
              frame Default {
                n148 = call <vilib>:"NT Read Number.vi"("Name"=w285) -> ("Numeric"=w286:dbl)  [unwired: 9 in, 1 out]
                n149 = call <vilib>:"NT Read String.vi"("Name"=w284) -> ("String"=w287:string)  [unwired: 9 in, 1 out]
                n150 = Bundle("Numeric"=w286, "String"=w287) -> (→"Progress":cluster{"Numeric":dbl, "String":string})  [unwired: 1 in]
              }
              frame "" {
                n151 = property on="Progress" class="Clust (strict)"("Visible"=FALSE) -> ()  [unwired: 2 in, 2 out]
                n152 = local write "Test Name"(u16 0) -> ()
              }
            }
            n153 = property on="Test Tree" class="Tree (strict)"("Active Item Row Number"=w281, "ActiveColNum"=w281, "CellBG"=w278, "Active Item Row Number"=-1 ("Active Item:Row Number"), "CellBG"=u32 5789784 ("Color Box")) -> ()  [unwired: 2 in, 2 out]
          }
          frame "Variables" {
            n154 = control-ref of="Tree"() -> (w292:refnum<vi>)
            n155 = call <vilib>:"NT Read and Format Entries as Tree.vi"("Operation"=enum16{"Update", "Clear"}."Update", "Tree Refnum"=w292) -> ()  [unwired: 8 in, 2 out]
          }
          frame "Commands" {
            w301 = u32 5789784 ("Color Box")
            w302 = T25 {"Row"=-1, "Column"=-2} ("Active Cell:Active Cell")
            w304 = T25 {"Row"=-2, "Column"=-2} ("Active Cell:Active Cell")
            n156 = Index Array(array=w305, index=w299) -> (element=w303:u32)
            n157 = Index Array(array=w300, index=w299) -> (element=w298:T24)
            n158 = Unbundle(w298) -> ("Operation"=w297:enum16{"Update", "Clear"})  [unwired: 1 out]
            n159 = local read "Command Selection"() -> (w296:i32)
            n160 = property on="Command Selection" class="MCListbox (strict)"("ActiveCell"=w304, "CellBG"=w303, "ActiveCell"=w302, "CellBG"=w301) -> ()  [unwired: 2 in, 2 out]
            n161 = call <vilib>:"WPI_DashboardUpdate RPC Info.vi"("Operation"=w297) -> ("update"=w295:bool, "commands"=w294:string[][])  [unwired: 9 in]
            n162 = property on="Command Selection" class="MCListbox (strict)"("ItemNames"=w294) -> ()  [unwired: 2 in, 2 out]
            n163 = property on="Command Params" class="Tbl (strict)"("Active Cell"=w304, "Cell BG Color"=w303, "Active Cell"=w302, "Cell BG Color"=w301) -> ()  [unwired: 2 in, 2 out]
            n164 = call <vilib>:"WPI_DashboardUpdate Command Params.vi"("Update"=w295, "NewVal"=w296, "Commands"=w294, "Param Tbl"=w293) -> ()  [unwired: 7 in, 1 out]
          }
        }
        n165 = case shown="\"Cam 2\"" "Camera Tab" {
          frame "Cam 1", Default {
          }
          frame "Cam 2" {
          }
          frame "Cam 3" {
          }
          frame "Graphs Setup" {
          }
          frame "Graphs" {
          }
        }
      }
      event "Test Tree": Value Change {
        # "Show appropriate\ncontrols"
        n166 = event-data() -> ("CtlRef"=w310:refnum<vi>, "NewVal"=w308:string)  [unwired: 1 in]
        n167 = call <vilib>:"WPI_UtilitiesGetTreeIOName.vi"("NewVal"=w308, "TreeControl in"=w310) -> ("I/O Name"=w311:string)  [unwired: 9 in]
        n168 = case shown="\"Camera\"" w311 {
          selector: w311 -> [_ w318 _ w340 w349 _]
          tunnel: w308 -> [_ _ w337 w339 _ w356]
          tunnel: cluster{string[]}[] [{["640x480", "320x240", "160x120"]}, {["Auto", "Fixed indoor", "Fixed outdoor 1", "Fixed outdoor 2", "Fixed fluorescent 1", "Fixed fluorescent 2", "Hold current"]}, {["Auto", "Flicker-free 50 Hz", "Flicker-free 60 Hz", "Hold current"]}, {["None", "Prioritize frame rate", "Prioritize image quality"]}, {["Monochrome", "Color"]}] -> [_ _ _ _ _ w355]
          frame Default {
            w313 = FALSE ("Visible")
            w312 = FALSE ("Visible")
            n169 = property on="Motor" class="Clust (strict)"("Visible"=w312) -> ()  [unwired: 2 in, 2 out]
            n170 = property on="Test Ring" class="Ring (strict)"("Visible"=w312) -> ()  [unwired: 2 in, 2 out]
            n171 = property on="Rev/Fwd" class="Clust (strict)"("Visible"=w313) -> ()  [unwired: 2 in, 2 out]
            n172 = property on="On/Off" class="Bool (strict)"("Visible"=w313) -> ()  [unwired: 2 in, 2 out]
            n173 = property on="Test Slider" class="Slide (strict)"("Visible"=w313) -> ()  [unwired: 2 in, 2 out]
          }
          frame "Analog Out", "Motor", "PWM" {
            w319 = FALSE ("Visible")
            n174 = case shown="\"Analog Out\"" w318 {
              tunnel: [1.0 ("Value") -1.0 ("Value") 0.0 ("Value")] -> w317
              tunnel: [255.0 ("Value") 1.0 ("Value") 5.0 ("Value")] -> w316
              tunnel: [128.0 ("Value") 0.0 ("Value") 0.0 ("Value")] -> w315
              tunnel: [64.0 ("Value") 0.5 ("Value") 1.0 ("Value")] -> w314
              frame "PWM" {
              }
              frame "Motor", Default {
              }
              frame "Analog Out" {
              }
            }
            n175 = property on="Motor" class="Clust (strict)"("Visible"=TRUE) -> ()  [unwired: 2 in, 2 out]
            n176 = property on="Value" class="Slide (strict)"("Value"=w315, "Scale.Minimum"=w317, "Scale.Maximum"=w316, "Scale.Increment"=w314) -> ()  [unwired: 2 in, 2 out]
            n177 = property on="On/Off" class="Bool (strict)"("Visible"=w319) -> ()  [unwired: 2 in, 2 out]
            n178 = property on="Test Slider" class="Slide (strict)"("Visible"=w319) -> ()  [unwired: 2 in, 2 out]
            n179 = property on="Test Ring" class="Ring (strict)"("Visible"=w319) -> ()  [unwired: 2 in, 2 out]
            n180 = property on="Rev/Fwd" class="Clust (strict)"("Visible"=w319) -> ()  [unwired: 2 in, 2 out]
          }
          frame "Servo" {
            w335 = FALSE ("Visible")
            n181 = call <vilib>:"NT Read Number.vi"("Name"=w337) -> ("Numeric"=w336:dbl)  [unwired: 9 in, 1 out]
            n182 = property on="Test Slider" class="Slide (strict)"("Visible"=TRUE, "Scale.Maximum"=170.0 ("Scale.Range:Maximum")) -> ()  [unwired: 2 in, 2 out]
            n183 = local write "Test Slider"(w336) -> ()
            n184 = property on="Motor" class="Clust (strict)"("Visible"=w335) -> ()  [unwired: 2 in, 2 out]
            n185 = property on="Rev/Fwd" class="Clust (strict)"("Visible"=w335) -> ()  [unwired: 2 in, 2 out]
            n186 = property on="On/Off" class="Bool (strict)"("Visible"=w335) -> ()  [unwired: 2 in, 2 out]
            n187 = property on="Test Ring" class="Ring (strict)"("Visible"=w335) -> ()  [unwired: 2 in, 2 out]
          }
          frame "Relay", "Solenoid" {
            w338 = FALSE ("Visible")
            n188 = property on="Motor" class="Clust (strict)"("Visible"=w338) -> ()  [unwired: 2 in, 2 out]
            n189 = property on="Test Slider" class="Slide (strict)"("Visible"=w338) -> ()  [unwired: 2 in, 2 out]
            n190 = Search and Replace String(input string=w339, search string="/Value  **", replace string="/Direction") -> (result string=w345:string)  [unwired: 5 in, 3 out]
            n191 = property on="Test Ring" class="Ring (strict)"("Visible"=w338) -> ()  [unwired: 2 in, 2 out]
            n192 = call <vilib>:"NT Read String.vi"("Name"=w345) -> ("String"=w343:string)  [unwired: 9 in, 1 out]
            n193 = Equal?(x="Both directions", y=w343) -> (x = y?=w341:bool)
            n194 = Not(x=w341) -> (.not. x?=w342:bool)
            n195 = property on="Rev/Fwd" class="Clust (strict)"("Visible"=w341) -> ()  [unwired: 2 in, 2 out]
            n196 = property on="On/Off" class="Bool (strict)"("Visible"=w342, "Caption.Text"=w340) -> ()  [unwired: 2 in, 2 out]
          }
          frame "Compressor", "Digital Out" {
            w348 = FALSE ("Visible")
            # "Get direction and finish"
            n197 = property on="Motor" class="Clust (strict)"("Visible"=w348) -> ()  [unwired: 2 in, 2 out]
            n198 = property on="Test Slider" class="Slide (strict)"("Visible"=w348) -> ()  [unwired: 2 in, 2 out]
            n199 = property on="Test Ring" class="Ring (strict)"("Visible"=w348) -> ()  [unwired: 2 in, 2 out]
            n200 = property on="On/Off" class="Bool (strict)"("Visible"=TRUE, "Caption.Text"=w349) -> ()  [unwired: 2 in, 2 out]
            n201 = property on="Rev/Fwd" class="Clust (strict)"("Visible"=FALSE) -> ()  [unwired: 2 in, 2 out]
          }
          frame "Camera" {
            n202 = call <vilib>:"Get Last Path Segment.vi"("String in"=w356) -> ("String out"=w357:string)  [unwired: 10 in]
            n203 = property on="On/Off" class="Bool (strict)"("Visible"=FALSE) -> ()  [unwired: 2 in, 2 out]
            n204 = property on="Motor" class="Clust (strict)"("Visible"=FALSE) -> ()  [unwired: 2 in, 2 out]
            n205 = property on="Rev/Fwd" class="Clust (strict)"("Visible"=FALSE) -> ()  [unwired: 2 in, 2 out]
            n206 = case shown="\"White Balance  **\"" w357 {
              tunnel: w356 -> [w363 w372 w381 w390 w399 _ w405]
              tunnel: w355 -> [w361 w369 w378 w387 w396 _ _]
              frame "Size  **" {
                n207 = Index Array(array=w361) -> (element=w360:cluster{string[]})  [unwired: 1 in]
                n208 = call <vilib>:"NT Read String.vi"("Name"=w363) -> ("String"=w362:string)  [unwired: 9 in, 1 out]
                n209 = Unbundle(w360) -> (w358:string[])
                n210 = Match First String(2:w358, 3:w362) -> (0:w359:i32)  [unwired: 1 out]
                n211 = property on="Test Ring" class="Ring (strict)"("Value"=w359, "Strings []"=w358) -> ()  [unwired: 2 in, 2 out]
                n212 = property on="Test Ring" class="Ring (strict)"("Visible"=TRUE) -> ()  [unwired: 2 in, 2 out]
                n213 = property on="Test Slider" class="Slide (strict)"("Visible"=FALSE) -> ()  [unwired: 2 in, 2 out]
              }
              frame "White Balance  **" {
                n214 = Index Array(array=w369, index=1) -> (element=w370:cluster{string[]})
                n215 = call <vilib>:"NT Read String.vi"("Name"=w372) -> ("String"=w371:string)  [unwired: 9 in, 1 out]
                n216 = Unbundle(w370) -> (w367:string[])
                n217 = Match First String(2:w367, 3:w371) -> (0:w366:i32)  [unwired: 1 out]
                n218 = property on="Test Ring" class="Ring (strict)"("Value"=w366, "Strings []"=w367) -> ()  [unwired: 2 in, 2 out]
                n219 = property on="Test Ring" class="Ring (strict)"("Visible"=TRUE) -> ()  [unwired: 2 in, 2 out]
                n220 = property on="Test Slider" class="Slide (strict)"("Visible"=FALSE) -> ()  [unwired: 2 in, 2 out]
              }
              frame "Exposure  **" {
                n221 = Index Array(array=w378, index=2) -> (element=w379:cluster{string[]})
                n222 = call <vilib>:"NT Read String.vi"("Name"=w381) -> ("String"=w380:string)  [unwired: 9 in, 1 out]
                n223 = Unbundle(w379) -> (w375:string[])
                n224 = Match First String(2:w375, 3:w380) -> (0:w376:i32)  [unwired: 1 out]
                n225 = property on="Test Ring" class="Ring (strict)"("Value"=w376, "Strings []"=w375) -> ()  [unwired: 2 in, 2 out]
                n226 = property on="Test Ring" class="Ring (strict)"("Visible"=TRUE) -> ()  [unwired: 2 in, 2 out]
                n227 = property on="Test Slider" class="Slide (strict)"("Visible"=FALSE) -> ()  [unwired: 2 in, 2 out]
              }
              frame "Exposure Priority  **" {
                n228 = Index Array(array=w387, index=3) -> (element=w388:cluster{string[]})
                n229 = call <vilib>:"NT Read String.vi"("Name"=w390) -> ("String"=w389:string)  [unwired: 9 in, 1 out]
                n230 = Unbundle(w388) -> (w384:string[])
                n231 = Match First String(2:w384, 3:w389) -> (0:w385:i32)  [unwired: 1 out]
                n232 = property on="Test Ring" class="Ring (strict)"("Value"=w385, "Strings []"=w384) -> ()  [unwired: 2 in, 2 out]
                n233 = property on="Test Ring" class="Ring (strict)"("Visible"=TRUE) -> ()  [unwired: 2 in, 2 out]
                n234 = property on="Test Slider" class="Slide (strict)"("Visible"=FALSE) -> ()  [unwired: 2 in, 2 out]
              }
              frame "Color Enable  **" {
                n235 = Index Array(array=w396, index=4) -> (element=w397:cluster{string[]})
                n236 = call <vilib>:"NT Read String.vi"("Name"=w399) -> ("String"=w398:string)  [unwired: 9 in, 1 out]
                n237 = Unbundle(w397) -> (w393:string[])
                n238 = Match First String(2:w393, 3:w398) -> (0:w394:i32)  [unwired: 1 out]
                n239 = property on="Test Ring" class="Ring (strict)"("Value"=w394, "Strings []"=w393) -> ()  [unwired: 2 in, 2 out]
                n240 = property on="Test Ring" class="Ring (strict)"("Visible"=TRUE) -> ()  [unwired: 2 in, 2 out]
                n241 = property on="Test Slider" class="Slide (strict)"("Visible"=FALSE) -> ()  [unwired: 2 in, 2 out]
              }
              frame Default {
                n242 = property on="Test Ring" class="Ring (strict)"("Visible"=FALSE) -> ()  [unwired: 2 in, 2 out]
                n243 = property on="Test Slider" class="Slide (strict)"("Visible"=FALSE) -> ()  [unwired: 2 in, 2 out]
              }
              frame "Brightness  **", "Color Level  **", "Compression  **", "FPS  **", "Sharpness  **" {
                n244 = call <vilib>:"NT Read Number.vi"("Name"=w405) -> ("Numeric"=w404:dbl)  [unwired: 9 in, 1 out]
                n245 = local write "Test Slider"(w404) -> ()
                n246 = property on="Test Slider" class="Slide (strict)"("Visible"=TRUE, "Scale.Maximum"=100.0 ("Scale.Range:Maximum")) -> ()  [unwired: 2 in, 2 out]
                n247 = property on="Test Ring" class="Ring (strict)"("Visible"=FALSE) -> ()  [unwired: 2 in, 2 out]
              }
            }
          }
        }
        n248 = property on="Progress" class="Clust (strict)"("Visible"=FALSE) -> ()  [unwired: 2 in, 2 out]
      }
      event "Test Name": Mouse Enter {
        # "Populate the ring with the list of tests"
        n249 = event-data() -> ()  [unwired: 1 in, 1 out]
        n250 = call <vilib>:"NT Read String Array.vi"("Name"="/TestMode/TestList") -> ("String Array"=w413:string[])  [unwired: 9 in, 1 out]
        n251 = Build Array (concatenate)("Select the test to run...", w413) -> (w412:string[])
        n252 = property on="Test Name" class="Ring (strict)"("Strings []"=w412) -> ()  [unwired: 2 in, 2 out]
      }
      event "Test Name": Value Change {
        w415 = FALSE ("Visible")
        # "Tell the robot the test name to run"
        n253 = event-data() -> ("NewVal"=w419:u16)  [unwired: 1 in]
        n254 = property on="Test Name" class="Ring (strict)"() -> ("Strings []"=w420:string[])  [unwired: 2 in, 2 out]
        n255 = local write "Progress"(T7 {"Test Progress"=0, "Test Progress Text"=""} ("Progress")) -> ()
        n256 = Index Array(array=w420, index=w419) -> (element=w418:string)
        n257 = call <vilib>:"NT Write String.vi"("String"=w418, "Name"="/TestMode/TestName") -> ()  [unwired: 9 in, 1 out]
        n258 = property on="Progress" class="Clust (strict)"("Visible"=TRUE) -> ()  [unwired: 2 in, 2 out]
        n259 = property on="Motor" class="Clust (strict)"("Visible"=w415) -> ()  [unwired: 2 in, 2 out]
        n260 = property on="Test Slider" class="Slide (strict)"("Visible"=w415) -> ()  [unwired: 2 in, 2 out]
        n261 = property on="On/Off" class="Bool (strict)"("Visible"=w415) -> ()  [unwired: 2 in, 2 out]
        n262 = property on="Rev/Fwd" class="Clust (strict)"("Visible"=w415) -> ()  [unwired: 2 in, 2 out]
        n263 = property on="Test Ring" class="Ring (strict)"("Visible"=w415) -> ()  [unwired: 2 in, 2 out]
      }
      event "Select Auto": Mouse Enter {
        # "Populate the combo box with the list of autonomous options"
        n264 = event-data() -> ()  [unwired: 1 in, 1 out]
        n265 = call <vilib>:"NT Read String Array.vi"("Name"="Auto List") -> ("String Array"=w422:string[])  [unwired: 9 in, 1 out]
        n266 = property on="Select Auto" class="CmbBox"("Strings[]"=w422) -> ()  [unwired: 2 in, 2 out]
      }
      event "Select Auto": Value Change {
        # "User modified the Auto Selection. Write to NT variable so robot knows."
        n267 = event-data() -> ("NewVal"=w425:string)  [unwired: 1 in]
        n268 = call <vilib>:"NT Write String.vi"("String"=w425, "Name"="Auto Selector") -> ()  [unwired: 9 in, 1 out]
      }
      event "Select Test": Mouse Enter {
        n269 = event-data() -> ()  [unwired: 1 in, 4 out]
        n270 = call-poly <vilib>:"NT Read Value.vi"("Name"="Test List") -> ("String Array"=w428:string[])  [unwired: 9 in, 1 out]
        n271 = property on="Select Test" class="CmbBox"("Strings[]"=w428) -> ()  [unwired: 2 in, 2 out]
      }
      event "Select Test": Value Change {
        n272 = event-data() -> ("NewVal"=w431:string)  [unwired: 1 in]
        n273 = call-poly <vilib>:"NT Write Value.vi"("String"=w431, "Name"="Test Selector") -> ()  [unwired: 9 in, 1 out]
      }
      event "Command Selection": Value Change {
        # "Get the params and show in table"
        n274 = event-data() -> ("NewVal"=w437:i32)  [unwired: 1 in]
        n275 = property on="Command Selection" class="MCListbox (strict)"() -> ("ItemNames"=w435:string[][])  [unwired: 2 in, 2 out]
        n276 = call <vilib>:"WPI_DashboardUpdate Command Params.vi"("NewVal"=w437, "Commands"=w435, "Param Tbl"=w436) -> ()  [unwired: 8 in, 1 out]
      }
      event "Execute Command": Value Change {
        # "Started one, Unique ID holds\nresponse"
        n277 = event-data() -> ()  [unwired: 1 in, 1 out]
        n278 = property on="Command Selection" class="MCListbox (strict)"() -> ("ItemNames"=w448:string[][])  [unwired: 2 in, 2 out]
        n279 = Index Array(array=w448, index (row)="Command Selection", index (col)=0) -> (element=w446:string)
        n280 = call <vilib>:"Invoke Commands.vi"("Command Params"="Command Params", "Function Name"=w446) -> ("Params"=w442:u8, "Started"=w441:bool)  [unwired: 7 in, 1 out]
        n281 = Array Subset(array="Command Params", length (row)=w442) -> (w443:string[][])  [unwired: 3 in]
        n282 = Select(t="Executing" ("Cmd Status"), s=w441, f="" ("Cmd Status")) -> (s? t:f=→"Cmd Status":string)
      }
      event "Command Selection": Double Click {
        n283 = event-data() -> ("Row"=w456:i32)  [unwired: 1 in]
        n284 = property on="Command Selection" class="MCListbox (strict)"() -> ("ItemNames"=w459:string[][])  [unwired: 2 in, 2 out]
        n285 = local read "Command Params"() -> (w455:string[][])
        n286 = Index Array(array=w459, index (row)=w456, index (col)=0) -> (element=w457:string)
        n287 = call <vilib>:"Invoke Commands.vi"("Command Params"=w455, "Function Name"=w457) -> ("Params"=w454:u8, "Started"=w449:bool)  [unwired: 7 in, 1 out]
        n288 = Array Subset(array=w455, length (row)=w454) -> (w453:string[][])  [unwired: 3 in]
        n289 = Select(t="Executing" ("Cmd Status"), s=w449, f="" ("Cmd Status")) -> (s? t:f=w450:string)
        n290 = local write "Cmd Status"(w450) -> ()
      }
      event "CheckList": Double Click {
        # "Shift clears all"
        # "Update symbols on the listbox"
        n291 = event-data() -> ("PlatMods.Shift"=w461:bool, "Row"=w463:i32)  [unwired: 1 in]
        n292 = case shown="True" w461 {
          tunnel: w463 -> [w467 _]
          tunnel: 1 -> [w466 _]
          frame False {
            n293 = property on="CheckList" class="LstBox (strict)"() -> ("Item Symbols"=w465:i32[])  [unwired: 2 in, 2 out]
            n294 = Replace Array Subset(array=w465, new element=w466, index=w467) -> (w464:i32[])
            n295 = property on="CheckList" class="LstBox (strict)"("Item Symbols"=w464) -> ()  [unwired: 2 in, 2 out]
          }
          frame True {
            w468 = 0 ("Top Row")
            n296 = property on="CheckList" class="LstBox (strict)"() -> ("Number of Rows"=w470:u32)  [unwired: 2 in, 2 out]
            n297 = Initialize Array(0, w470) -> (w469:i32[])
            n298 = property on="CheckList" class="LstBox (strict)"("Top Row"=w468, "Value"=w468, "Item Symbols"=w469) -> ()  [unwired: 2 in, 2 out]
          }
        }
      }
      event "CheckList": Key Down {
        # "Update symbols on the listbox\nLeft and right keys check and uncheck"
        n299 = event-data() -> ("VKey"=w474:T22)  [unwired: 1 in]
        n300 = case shown="\"Left\", \"Right\"" w474 {
          selector: w474 -> [w479 _]
          tunnel: eventvkey."Left" ("VKey") -> [w477 _]
          frame "Left", "Right" {
            n301 = Equal?(x=w477, y=w479) -> (x = y?=w478:bool)
            n302 = Select(t=0, s=w478, f=1) -> (s? t:f=w480:i32)
            n303 = property on="CheckList" class="LstBox (strict)"() -> ("Item Symbols"=w483:i32[])  [unwired: 2 in, 2 out]
            n304 = Replace Array Subset(array=w483, new element=w480, index="CheckList") -> (w482:i32[])
            n305 = property on="CheckList" class="LstBox (strict)"("Item Symbols"=w482) -> ()  [unwired: 2 in, 2 out]
          }
          frame Default {
          }
        }
      }
      event "Motor.Enable": Value Change {
        # "When the test mode otor enable helper is set, update that\ntree row item's value"
        n306 = event-data() -> ("NewVal"=w489:bool)  [unwired: 1 in]
        n307 = Unbundle("Motor") -> ("Value"=w488:dbl)  [unwired: 1 out]
        n308 = Select(t=w488, s=w489, f=0.0) -> (s? t:f=w486:dbl)
        n309 = call <vilib>:"NT Write Number.vi"("Numeric"=w486, "Name"=w485) -> ()  [unwired: 9 in, 1 out]
      }
      event "Test Slider": Value Change {
        # "When the test mode slider helper is set, update that\ntree row item's value"
        n310 = event-data() -> ("NewVal"=w492:dbl)  [unwired: 1 in]
        n311 = call <vilib>:"NT Write Number.vi"("Numeric"=w492, "Name"=w493) -> ()  [unwired: 9 in, 1 out]
      }
      event "On/Off": Value Change {
        # "When the test mode on/off helper value is set, update that\ntree row item's value"
        n312 = event-data() -> ("NewVal"=w497:bool)  [unwired: 1 in]
        n313 = Boolean To (0,1)(Boolean=w497) -> (0, 1=w496:i16)
        n314 = call <vilib>:"NT Write Number.vi"("Numeric"=w496, "Name"=w495) -> ()  [unwired: 9 in, 1 out]
      }
      event "Rev/Fwd": Value Change {
        # "When the test mode helper value for relays is set, update that\ntree row item's value"
        n315 = event-data() -> ("NewVal.Forward"=w505:bool, "NewVal.Reverse"=w504:bool)  [unwired: 1 in]
        n316 = Boolean To (0,1)(Boolean=w505) -> (0, 1=w501:i16)
        n317 = Boolean To (0,1)(Boolean=w504) -> (0, 1=w503:i16)
        n318 = Negate(x=w503) -> (-x=w502:i16)
        n319 = Add(x=w501, y=w502) -> (x+y=w500:i16)
        n320 = call <vilib>:"NT Write Number.vi"("Numeric"=w500, "Name"=w499) -> ()  [unwired: 9 in, 1 out]
      }
      event "Test Ring": Value Change {
        # "When a test mode helper value is selected from the ring,\nset the tree item's variable to the string value"
        n321 = event-data() -> ("NewVal"=w509:u16)  [unwired: 1 in]
        n322 = property on="Test Ring" class="Ring (strict)"() -> ("Strings []"=w510:string[])  [unwired: 2 in, 2 out]
        n323 = Index Array(array=w510, index=w509) -> (element=w508:string)
        n324 = call <vilib>:"NT Write String.vi"("String"=w508, "Name"=w507) -> ()  [unwired: 9 in, 1 out]
      }
      event "Rec Mode": Value Change {
        # "Update globals for recording mode and path to read log from.\nClear when logging and let NetworkTables set path for vision to\nuse."
        n325 = event-data() -> ("NewVal"=w521:enum32{"Stop", "Record", "Playback"})  [unwired: 1 in]
        n326 = global write "WPI_DashboardLogging Global.vi" "Logging Filename"(path "") -> ()
        n327 = global write "WPI_DashboardLogging Global.vi" "Recording"(w521) -> ()
        n328 = case shown="\"Playback\"" w521 {
          tunnel: w520 -> [_ w523 w532]
          tunnel: [_ _ w531] -> w518
          tunnel: [_ _ w530] -> _
          tunnel: w516 -> [_ _ w528]
          tunnel: cluster{i32, i32} {-250, 170} -> [_ _ w527]
          tunnel: [_ _ T23 {"Image Size"=TRUE, "Image Type"=TRUE, "Pixel Value"=TRUE, "ROI Information"=TRUE, "Zoom Factor"=FALSE} ("Image Information Shown:All Elements")] -> w514
          tunnel: [_ _ TRUE ("Zoom Factor")] -> w513
          tunnel: w512 -> [_ _ w524]
          frame Default {
          }
          frame "Stop", "Record" {
            # "Place Window too"
            n329 = invoke class="VI" method="FP.Close"(reference=w523) -> (reference out=w522:refnum<vi>)  [unwired: 2 in, 2 out]
            n330 = invoke class="VI" method="Abort VI"(reference=w522) -> ()  [unwired: 2 in, 3 out]
          }
          frame "Playback" {
            n331 = call "Open Playback Panel.vi"("Offset"=w527, "DB VI Ref"=w528, "Playback in"=w532) -> ("Playback out"=w529:refnum<vi>)  [unwired: 8 in]
            n332 = register-events(w529, w524) -> (reference out=w531:refnum<event-registration>, error out=w530:errorcluster)  [unwired: 2 in]
          }
        }
        n333 = property on="Dashboard Image 1" class="ImageControl"("Image Information Shown"=w514, "Image Information Visible"=w513) -> ()  [unwired: 2 in, 2 out]
        n334 = call <vilib>:"WPI_DashboardNT Log FieldName Cache.vi"("Operation"=enum16{"Lookup/Add", "Index", "Clear"}."Clear") -> ()  [unwired: 8 in, 3 out]
      }
      event Panel Close {
        w534 = enum32{"Stop", "Record", "Playback"}."Stop" ("Rec Mode")
        # "Playback window has been closed, abort"
        n335 = event-data() -> ()  [unwired: 1 in, 4 out]
        n336 = local write "Rec Mode"(w534) -> ()
        n337 = global write "WPI_DashboardLogging Global.vi" "Recording"(w534) -> ()
      }
      event Panel Close {
        # "Abort playback window and ourself"
        n338 = event-data() -> ()  [unwired: 1 in, 4 out]
        n339 = invoke class="VI" method="FP.Close"(reference=w538) -> (reference out=w537:refnum<vi>)  [unwired: 2 in, 2 out]
        n340 = invoke class="VI" method="Abort VI"(reference=w537) -> (error out=w536:errorcluster)  [unwired: 2 in, 2 out]
        n341 = invoke class="VI" method="Abort VI"(error in=w536) -> ()  [unwired: 2 in, 3 out]
      }
      event User Event {
        n342 = event-data() -> ("IDs"=w545:cluster{"RPC field ID":u16, "Unique ID":u16}, "String"=w544:string)  [unwired: 1 in]
        n343 = Bundle("IDs"=w545, "String"=w544) -> (w543:T9)  [unwired: 1 in]
        n344 = call <vilib>:"Retrieve RPC Response.vi"("RPC Response"=w543) -> ("Output"=w541:string[][])  [unwired: 10 in]
        n345 = Build Array (concatenate)(w539, w541) -> (w540:string[][])
        n346 = local write "Command Params"(w540) -> ()
        n347 = local write "Cmd Status"("" ("Cmd Status")) -> ()
      }
      event "Camera Tab": Mouse Enter {
        n348 = event-data() -> ()  [unwired: 1 in, 4 out]
        n349 = property on="Tree" class="Tree (strict)"() -> ("All Tags"=w546:string[])  [unwired: 2 in, 2 out]
        n350 = for {
          tunnel: w546 -> [w556] mode=indexing
          tunnel: [w556] -> w547 mode=indexing if=w554
          n351 = Empty String/Path?(string/path="Graph Include Filter") -> (empty?=w552:bool[])
          n352 = property on="Tree" class="Tree (strict)"("Active Item Tag"=w556, "ActiveColNum"=2 ("Active Cell:Active Column Number")) -> ("Cell String"=w562:string)  [unwired: 2 in, 2 out]
          n353 = And Array Elements(Boolean array=w552) -> (logical AND=w551:bool)
          n354 = case shown="False" w551 {
            selector: w551 -> [_ w573]
            tunnel: w556 -> [w566 _]
            tunnel: [w565 w573] -> w555
            tunnel: "Graph Include Filter" -> [w564 _]
            frame False {
              n355 = for {
                tunnel: [w572] -> w567 mode=indexing
                tunnel: w564 -> [w570] mode=indexing
                tunnel: w566 -> [w569]
                n356 = Match Pattern(string=w569, regular expression=w570) -> (match substring=w571:string)  [unwired: 1 in, 3 out]
                n357 = Empty String/Path?(string/path=w571) -> (empty?=w572:bool)
              }
              n358 = Not(x=w567) -> (.not. x?=w568:bool[])
              n359 = Or Array Elements(Boolean array=w568) -> (logical OR=w565:bool)
            }
            frame True {
            }
          }
          n360 = for {
            tunnel: "Graph Exclude Filter" -> [w577] mode=indexing
            tunnel: w556 -> [w575]
            tunnel: [w576] -> w558 mode=indexing
            n361 = Match Pattern(string=w575, regular expression=w577) -> (match substring=w574:string)  [unwired: 1 in, 3 out]
            n362 = Empty String/Path?(string/path=w574) -> (empty?=w576:bool)
          }
          n363 = Equal?(x="Numeric" ("y"), y=w562) -> (x = y?=w559:bool)
          n364 = And Array Elements(Boolean array=w558) -> (logical AND=w557:bool)
          n365 = Compound Arithmetic op=AND(w559, w557, w555) -> (w554:bool)
        }
        n366 = Build Array (concatenate)("Select Variable", w547) -> (w549:string[])
        n367 = property on="Combo Box" class="CmbBox"("Strings[]"=w549) -> ()  [unwired: 2 in, 2 out]
        n368 = property on="Combo Box 2" class="CmbBox"("Strings[]"=w549) -> ()  [unwired: 2 in, 2 out]
        n369 = property on="Combo Box 3" class="CmbBox"("Strings[]"=w549) -> ()  [unwired: 2 in, 2 out]
        n370 = property on="Combo Box 4" class="CmbBox"("Strings[]"=w549) -> ()  [unwired: 2 in, 2 out]
        n371 = property on="Combo Box 5" class="CmbBox"("Strings[]"=w549) -> ()  [unwired: 2 in, 2 out]
        n372 = property on="Combo Box 6" class="CmbBox"("Strings[]"=w549) -> ()  [unwired: 2 in, 2 out]
        n373 = property on="Combo Box 7" class="CmbBox"("Strings[]"=w549) -> ()  [unwired: 2 in, 2 out]
        n374 = property on="Combo Box 8" class="CmbBox"("Strings[]"=w549) -> ()  [unwired: 2 in, 2 out]
      }
      event "Tree": Double Click {
        n375 = event-data() -> ("PlatMods"=w581:T26, "Tag"=w580:string)  [unwired: 1 in]
        n376 = Unbundle(w581) -> ("Shift"=w579:bool)  [unwired: 4 out]
        n377 = Not(x=w579) -> (.not. x?=w578:bool)
        n378 = call <vilib>:"NT Update Persistence.vi"("Persistence"=w578, "Name"=w580) -> ()  [unwired: 9 in, 1 out]
      }
    }
  }
  n379 = while {
    tunnel: w73 -> [w584]
    i -> [w587]
    stop <- FALSE stop-if-true
    n380 = Wait (ms)(milliseconds to wait=u32 100) -> ()  [unwired: 1 out]
    n381 = case shown="\"Playback\"" "Rec Mode" {
      tunnel: w587 -> [_ _ w602]
      tunnel: [u32 2829099 ("Base Color") u32 11141120 ("Target Color") w591] -> w583
      frame "Stop", Default {
        # "Reset the color, extra updates don't cost much"
      }
      frame "Record" {
      }
      frame "Playback" {
        # "Playback"
        n382 = Quotient & Remainder(x=w602, y=u32 50 ("milliseconds to wait")) -> (x-y*floor(x/y)=w598:u32)  [unwired: 1 out]
        n383 = Divide(x=w598, y=u32 50 ("milliseconds to wait")) -> (x/y=w595:dbl)
        n384 = Multiply(x=6.283185307179586, y=w595) -> (x*y=w600:dbl)
        n385 = Sine(x=w600) -> (sin(x)=w599:dbl)
        n386 = Absolute Value(x=w599) -> (abs(x)=w592:dbl)
        n387 = call "Interpolate RGB Color.vi"("Proportion"=w592, "Target Color"=u32 30976, "Base Color"=u32 2829099) -> ("Result Color"=w591:u32)  [unwired: 8 in]
      }
    }
    n388 = property class="Pane"(reference=w584, "PaneColor"=w583) -> ()  [unwired: 1 in, 2 out]
  }
  n389 = local write "Dashboard Tab"(T4."Drive" ("Dashboard Tab")) -> ()
  n390 = property on="On/Off" class="Bool (strict)"("Visible"=w43) -> ()  [unwired: 2 in, 2 out]
  n391 = property on="Motor" class="Clust (strict)"("Visible"=w43) -> ()  [unwired: 2 in, 2 out]
  n392 = property on="Progress" class="Clust (strict)"("Visible"=w43) -> ()  [unwired: 2 in, 2 out]
  n393 = property on="Test Ring" class="Ring (strict)"("Visible"=w43) -> ()  [unwired: 2 in, 2 out]
  n394 = property on="Rev/Fwd" class="Clust (strict)"("Visible"=w43) -> ()  [unwired: 2 in, 2 out]
  n395 = while {
    tunnel: u16 1741 ("timeout ms (25000)") -> [w604]
    stop <- FALSE stop-if-true
    n396 = TCP Create Listener(10:w604) -> (0:w603:errorcluster, 3:w605:refnum<k5>)  [unwired: 4 in, 1 out]
    n397 = case shown="No Error" w603 {
      selector: w603 -> [w607 _]
      tunnel: w605 -> [w608 _]
      frame No Error {
        n398 = while {
          tunnel: w608 -> [w611]
          tunnel: w607 -> [w610]
          stop <- FALSE stop-if-true
          n399 = TCP Wait On Listener(8:w610, 11:w611) -> (0:w612:errorcluster, 4:w613:refnum<k5>)  [unwired: 2 in, 3 out]
          n400 = local write "TCP"(w613) -> ()
          n401 = case shown="No Error" w612 {
            frame No Error {
            }
            frame Error {
              n402 = Wait (ms)(milliseconds to wait=u32 1000) -> ()  [unwired: 1 out]
            }
          }
        }
      }
      frame Error {
        n403 = Wait (ms)(milliseconds to wait=u32 1000) -> ()  [unwired: 1 out]
      }
    }
  }
  n404 = local write "Command Selection"(u16 0 ("milliseconds to wait")) -> ()
  n405 = local write "Command Params"(string[][] [] ("Command Params")) -> ()
  n406 = global write "WPI_DashboardLogging Global.vi" "Recording"(w67) -> ()
  n407 = local write "Rec Mode"(w67) -> ()
  n408 = invoke on="Waveform Chart" class="WFChart (strict)" method="Reinit To Default"() -> (error out=w2:errorcluster)  [unwired: 3 in, 2 out]
  n409 = invoke on="Waveform Chart 2" class="WFChart (strict)" method="Reinit To Default"() -> (error out=w1:errorcluster)  [unwired: 3 in, 2 out]
  n410 = property on="Waveform Chart 2" class="WFChart (strict)"(error in=w1, "Value"=w4, "XScale.Range"=w3) -> (error out=w5:errorcluster)  [unwired: 1 in, 1 out]
  n411 = property on="Waveform Chart" class="WFChart (strict)"(error in=w2, "Value"=w4, "XScale.Range"=w3) -> (error out=w6:errorcluster)  [unwired: 1 in, 1 out]
  n412 = disable-structure shown="Enabled" {
    frame Enabled {
      w621 = T11 4 items=["Grayscale (U8)", "Grayscale (I16)", "Grayscale (SGL)", "Complex (CSG)", "RGB (U32)", "HSL (U32)", "RGB (U64)"] ("Image Type")
      n413 = call "IMAQ Create"("Image Name"="Dashboard Image 3", "Image Type"=w621) -> ("New Image"=w620:T3, "error out"=w619:errorcluster)  [unwired: 2 in, 1 out]
      n414 = while {
        tunnel: w620 -> [w630]
        tunnel: w619 -> [_]
        stop <- FALSE stop-if-true
        n415 = local read "Robot IP"() -> (w632:string)
        n416 = local read "Rec Mode"() -> (w633:enum32{"Stop", "Record", "Playback"})
        n417 = call <vilib>:"WPI_CameraRead MJPG for Dashboard.vi"("Camera Settings"="Camera Settings 3", "Rec Mode"=w633, "Robot IP"=w632, "Camera Name"="Camera Name 3", "Refnum in"=w630) -> ("Active"=w625:bool, "Refnum out"=w627:T3, "FPS"=w626:dbl, "Bandwidth (Mbps)"=w628:dbl)  [unwired: 3 in]
        n418 = case shown="True" w625 {
          tunnel: w627 -> [w637 w647]
          tunnel: w628 -> [_ w643]
          tunnel: w626 -> [_ w648]
          tunnel: [w637 w646] -> w623
          frame False {
            w636 = u32 1985280 ("Color Box")
            n419 = Bundle("Color Box"=w636, "Color Box"=w636) -> (w635:cluster{"Color Box":u32, "Color Box":u32})  [unwired: 1 out]
            n420 = Wait Until Next ms Multiple(millisecond multiple=u32 500) -> ()  [unwired: 1 out]
            n421 = Build Array(w635) -> (w634:cluster{"Color Box":u32, "Color Box":u32}[])
            n422 = property on="Mbps LED" class="Bool (strict)"("Colors [4]"=w634) -> ()  [unwired: 2 in, 2 out]
          }
          frame True {
            n423 = case shown="Default" w643 {
              tunnel: [u32 6618880 ("Color Box") u32 16776722 ("Color Box") u32 16716800 ("Color Box")] -> w641
              frame Default {
              }
              frame 4, 5 {
              }
              frame 6.. {
              }
            }
            n424 = Bundle(FALSE, "Bandwidth (Mbps)"=w643, "FPS"=w648) -> (→"Camera Info 3":cluster{bool, "Bandwidth (Mbps)":dbl, "FPS":dbl})  [unwired: 1 in]
            n425 = call "IMAQ Clear Overlay"("Image"=w647) -> ("error out"=w645:errorcluster, "Image Out"=w646:T3)  [unwired: 2 in, 7 out]
            n426 = Unbundle By Name(w645) -> ("status"=w644:bool)
            n427 = Bundle("Color Box"=w641, "Color Box"=w641) -> (w642:cluster{"Color Box":u32, "Color Box":u32})  [unwired: 1 out]
            n428 = Build Array(w642) -> (w640:cluster{"Color Box":u32, "Color Box":u32}[])
            n429 = property on="Image Message 3" class="Str"("Visible"=w644) -> ()  [unwired: 2 in, 2 out]
            n430 = property on="Mbps LED" class="Bool (strict)"("Colors [4]"=w640) -> ()  [unwired: 2 in, 2 out]
          }
        }
        "Dashboard Image 3" <- w623
        "Image 3" <- w623
      }
      n431 = control-ref of="Camera Settings 3"() -> (w617:refnum<vi>)
      n432 = control-ref of="Camera Name 3"() -> (w616:refnum<vi>)
      n433 = call "Handle Camera Configuration.vi"("CameraNameRef"=w616, "Camera File Name"="Cam3", "ClusterRef"=w617) -> ()  [unwired: 9 in]
    }
    frame Disabled {
    }
  }
  n434 = node-c288() -> (w15:T27)  [unwired: 3 in]
  n435 = timed-loop {
    timing: w15 -> [_]
    timing-out: [_] -> w14
    shift-right: [w666] -> _
    shift-left: dbl[] [] -> [w667]
    tunnel: w6 -> [_]
    tunnel: w5 -> [_]
    shift-right: [w656] -> _
    shift-left: _ -> [w658]
    i -> [w663]
    stop <- FALSE stop-if-true
    w676 = "Select Variable"
    n436 = node-c288() -> (w670:i64)  [unwired: 1 in, 2 out]
    n437 = Array Size(array=w667) -> (size(s)=w664:i32)
    n438 = Greater?(x=w664, y="# Samples") -> (0:w665:bool)
    n439 = Build Array("Combo Box 5", "Combo Box 6", "Combo Box 7", "Combo Box 8") -> (w677:string[])
    n440 = Build Array("Combo Box", "Combo Box 2", "Combo Box 3", "Combo Box 4") -> (w683:string[])
    n441 = To Double Precision Float(number=w670) -> (double precision float=w671:dbl)
    n442 = Divide(x=w671, y=1000000000.0) -> (x/y=w668:dbl)
    n443 = for {
      tunnel: w683 -> [w710] mode=indexing
      tunnel: w676 -> [w711]
      tunnel: [w710] -> w682 mode=indexing if=w712
      n444 = Not Equal?(x=w710, y=w711) -> (x != y?=w712:bool)
    }
    n445 = for {
      tunnel: w677 -> [w708] mode=indexing
      tunnel: w676 -> [w709]
      tunnel: [w708] -> w675 mode=indexing if=w707
      n446 = Not Equal?(x=w709, y=w708) -> (x != y?=w707:bool)
    }
    n447 = case shown="True" w665 {
      tunnel: w668 -> [w699 w703]
      tunnel: w667 -> [w698 w702]
      tunnel: [w697 w704] -> w666
      frame False {
        n448 = Build Array (concatenate)(w699, w698) -> (w697:dbl[])
      }
      frame True {
        n449 = Array Subset(array=w702, index=1) -> (w701:dbl[])  [unwired: 1 in]
        n450 = Build Array (concatenate)(w703, w701) -> (w704:dbl[])
      }
    }
    n451 = for {
      tunnel: w682 -> [w714] mode=indexing
      tunnel: [w713] -> w659 mode=indexing
      n452 = call-poly <vilib>:"NT Read Value.vi"("Name"=w714) -> ("Numeric"=w713:dbl)  [unwired: 9 in, 1 out]
    }
    n453 = for {
      tunnel: w675 -> [w706] mode=indexing
      tunnel: [w705] -> w655 mode=indexing
      n454 = call-poly <vilib>:"NT Read Value.vi"("Name"=w706) -> ("Numeric"=w705:dbl)  [unwired: 9 in, 1 out]
    }
    n455 = Build Array(w655) -> (w654:dbl[][])
    n456 = case shown="False" "Pause" {
      tunnel: w654 -> [w687 _]
      frame False {
        "Waveform Chart 2" <- w687
      }
      frame True {
      }
    }
    n457 = Build Array (concatenate)(w659, w658) -> (w657:dbl[][])
    n458 = Quotient & Remainder(x=w663, y=10) -> (x-y*floor(x/y)=w661:i32)  [unwired: 1 out]
    n459 = Equal To 0?(x=w661) -> (x = 0?=w660:bool)
    n460 = case shown="True" w660 {
      tunnel: w657 -> [w688 w691]
      tunnel: [w688 w690] -> w656
      tunnel: "Pause" -> [_ w689]
      frame False {
      }
      frame True {
        n461 = case shown="False" w689 {
          tunnel: w691 -> [w693 w694]
          tunnel: [dbl[][] [] w694] -> w690
          frame False {
            "Waveform Chart" <- w693
          }
          frame True {
            n462 = property on="Waveform Chart" class="WFChart (strict)"() -> ("XScale.Minimum"=w695:dbl, "XScale.Maximum"=w696:dbl)  [unwired: 2 in, 2 out]
            n463 = property on="Waveform Chart 2" class="WFChart (strict)"("XScale.Minimum"=w695, "XScale.Maximum"=w696) -> ()  [unwired: 2 in, 2 out]
          }
        }
      }
    }
    n464 = node-c288() -> ()  [unwired: 1 in, 1 out]
  }
  n465 = while {
    stop <- FALSE stop-if-true
    n466 = property on="Get Data" class="Bool (strict)"() -> ("Label.Text"=w719:string)  [unwired: 2 in, 2 out]
    n467 = case shown="True" "Reset" {
      frame False {
      }
      frame True {
        w723 = dbl[][] [] ("History Data")
        n468 = invoke on="Waveform Chart" class="WFChart (strict)" method="ForceRedraw"() -> ()  [unwired: 3 in, 3 out]
        n469 = invoke on="Waveform Chart 2" class="WFChart (strict)" method="ForceRedraw"() -> ()  [unwired: 3 in, 3 out]
        n470 = property on="Waveform Chart" class="WFChart (strict)"("History Data"=w723) -> ()  [unwired: 2 in, 2 out]
        n471 = property on="Waveform Chart 2" class="WFChart (strict)"("History Data"=w723) -> ()  [unwired: 2 in, 2 out]
      }
    }
    n472 = call-poly <vilib>:"NT Write Value.vi"("Boolean"="Get Data", "Name"=w719) -> ()  [unwired: 9 in, 1 out]
    n473 = Wait Until Next ms Multiple(millisecond multiple=u32 250) -> ()  [unwired: 1 out]
  }
  n474 = node-c288(w14) -> ()  [unwired: 1 out]
